vi "DualSimpleLiveAppStreamSaving.vi"() -> ()   [LabVIEW 2020]
uses:
  C:/Users/Public/Documents/Photometrics/PMQI-LabViewSamples/Examples/2018/Dependencies/PVCamNET.dll
  Dependencies/PVCamNET.dll
panel:
  out "Multi Page TIFF Size Read 2":u64 max=1 step=1
  out "Multi Page TIFF Size Read":u64 max=1 step=1
  in  "Multi Page TIFF Size 2 [B]":u64 max=1 step=1
  out "Big TIFF 2":bool
  in  "Big TIFF On/Off 2":bool
  in  "Multi Page TIFF Size [B]":u64 max=1 step=1
  out "Big TIFF":bool
  in  "Big TIFF On/Off":bool
  in  "Trigger Out Behaviour 2":string(combo)
  in  "Trigger In Behaviour 2":string(combo)
  in  "Trigger Out Behaviour":string(combo)
  in  "Trigger In Behaviour":string(combo)
  in  "Live 3":bool
  out "Disk Streaming Queue Size 2":u64
  out "Dropped Frames 2":i32
  out "Buffer Index 2":i32
  in  "Path 2":path
  out "StreamSavingPath 2":string
  in  "Format 2":u8 max=1 step=1
  out "Stream Saving 2":bool
  in  "Stream Saving On/Off 2":bool
  in  "Exposure Time 2":dbl
  in  "Live 2":bool
  out "Available Ram":u64
  out "Disk Streaming Queue Size":u64
  out "Dropped Frames":i32
  out "Buffer Index":i32
  in  "Path":path
  out "StreamSavingPath":string
  in  "Format":u8 max=1 step=1
  out "Stream Saving":bool
  in  "Stream Saving On/Off":bool
  in  "Exposure Time":dbl
  in  "Live":bool
  in  "Camera Status":bool
  in  "Uninit":bool
  in  "Live stop":bool
  in  "Live start":bool
  in  "Init":bool
  # "DualSimpleLiveAppStreamSaving.vi\n\nDescription:\nThis sample code lets the user use \nstream saving and trigger in/out with live mode \nin an event driven structure.\n\nSteps to run:\n1. Connect two cameras. \n2. Click \"Run\"\n3. Click \"Open\" to open two cameras\n4. Enter Exposure Time\n5. Turn On/Off display\n6. Toggle Big TIFF\n7. Enter multi page TIFF size (at default the staxk size is 2GB for regular TIFF and 4GB for Big TIFF)\n8. Select the path for images to be saved at\n9. Turn \"On\" Stream Saving\n10. Click \"Live start\"\n11. Click \"Live stop\"\n12. Click \"Close\""
  # "Camera 1"
  # "Camera 2"
  # "Note about Tiff and BigTiff saving:\n\n\tAt default images are stored with regular Tiff and the maximum multi-image size is 2GB.\n\nIf you would like to save 6GB with Big Tiff then\n    BIG TIFF ON /OFF = ON;\n    Multi Page TIFF Size = 6442450944; (in bytes)\n\t\t\nIfyou would like to save 1 page per file with regular Tiff\n    BIG TIFF ON /OFF = ON;\n    Multi Page TIFF Size =1; (any number smaller than a frame size except 0)\n\t\t\nIf you would like to save 2GB with regular Tiff then\n    BIG TIFF ON /OFF = OFF;\n    Multi Page TIFF Size = 2147483648;"
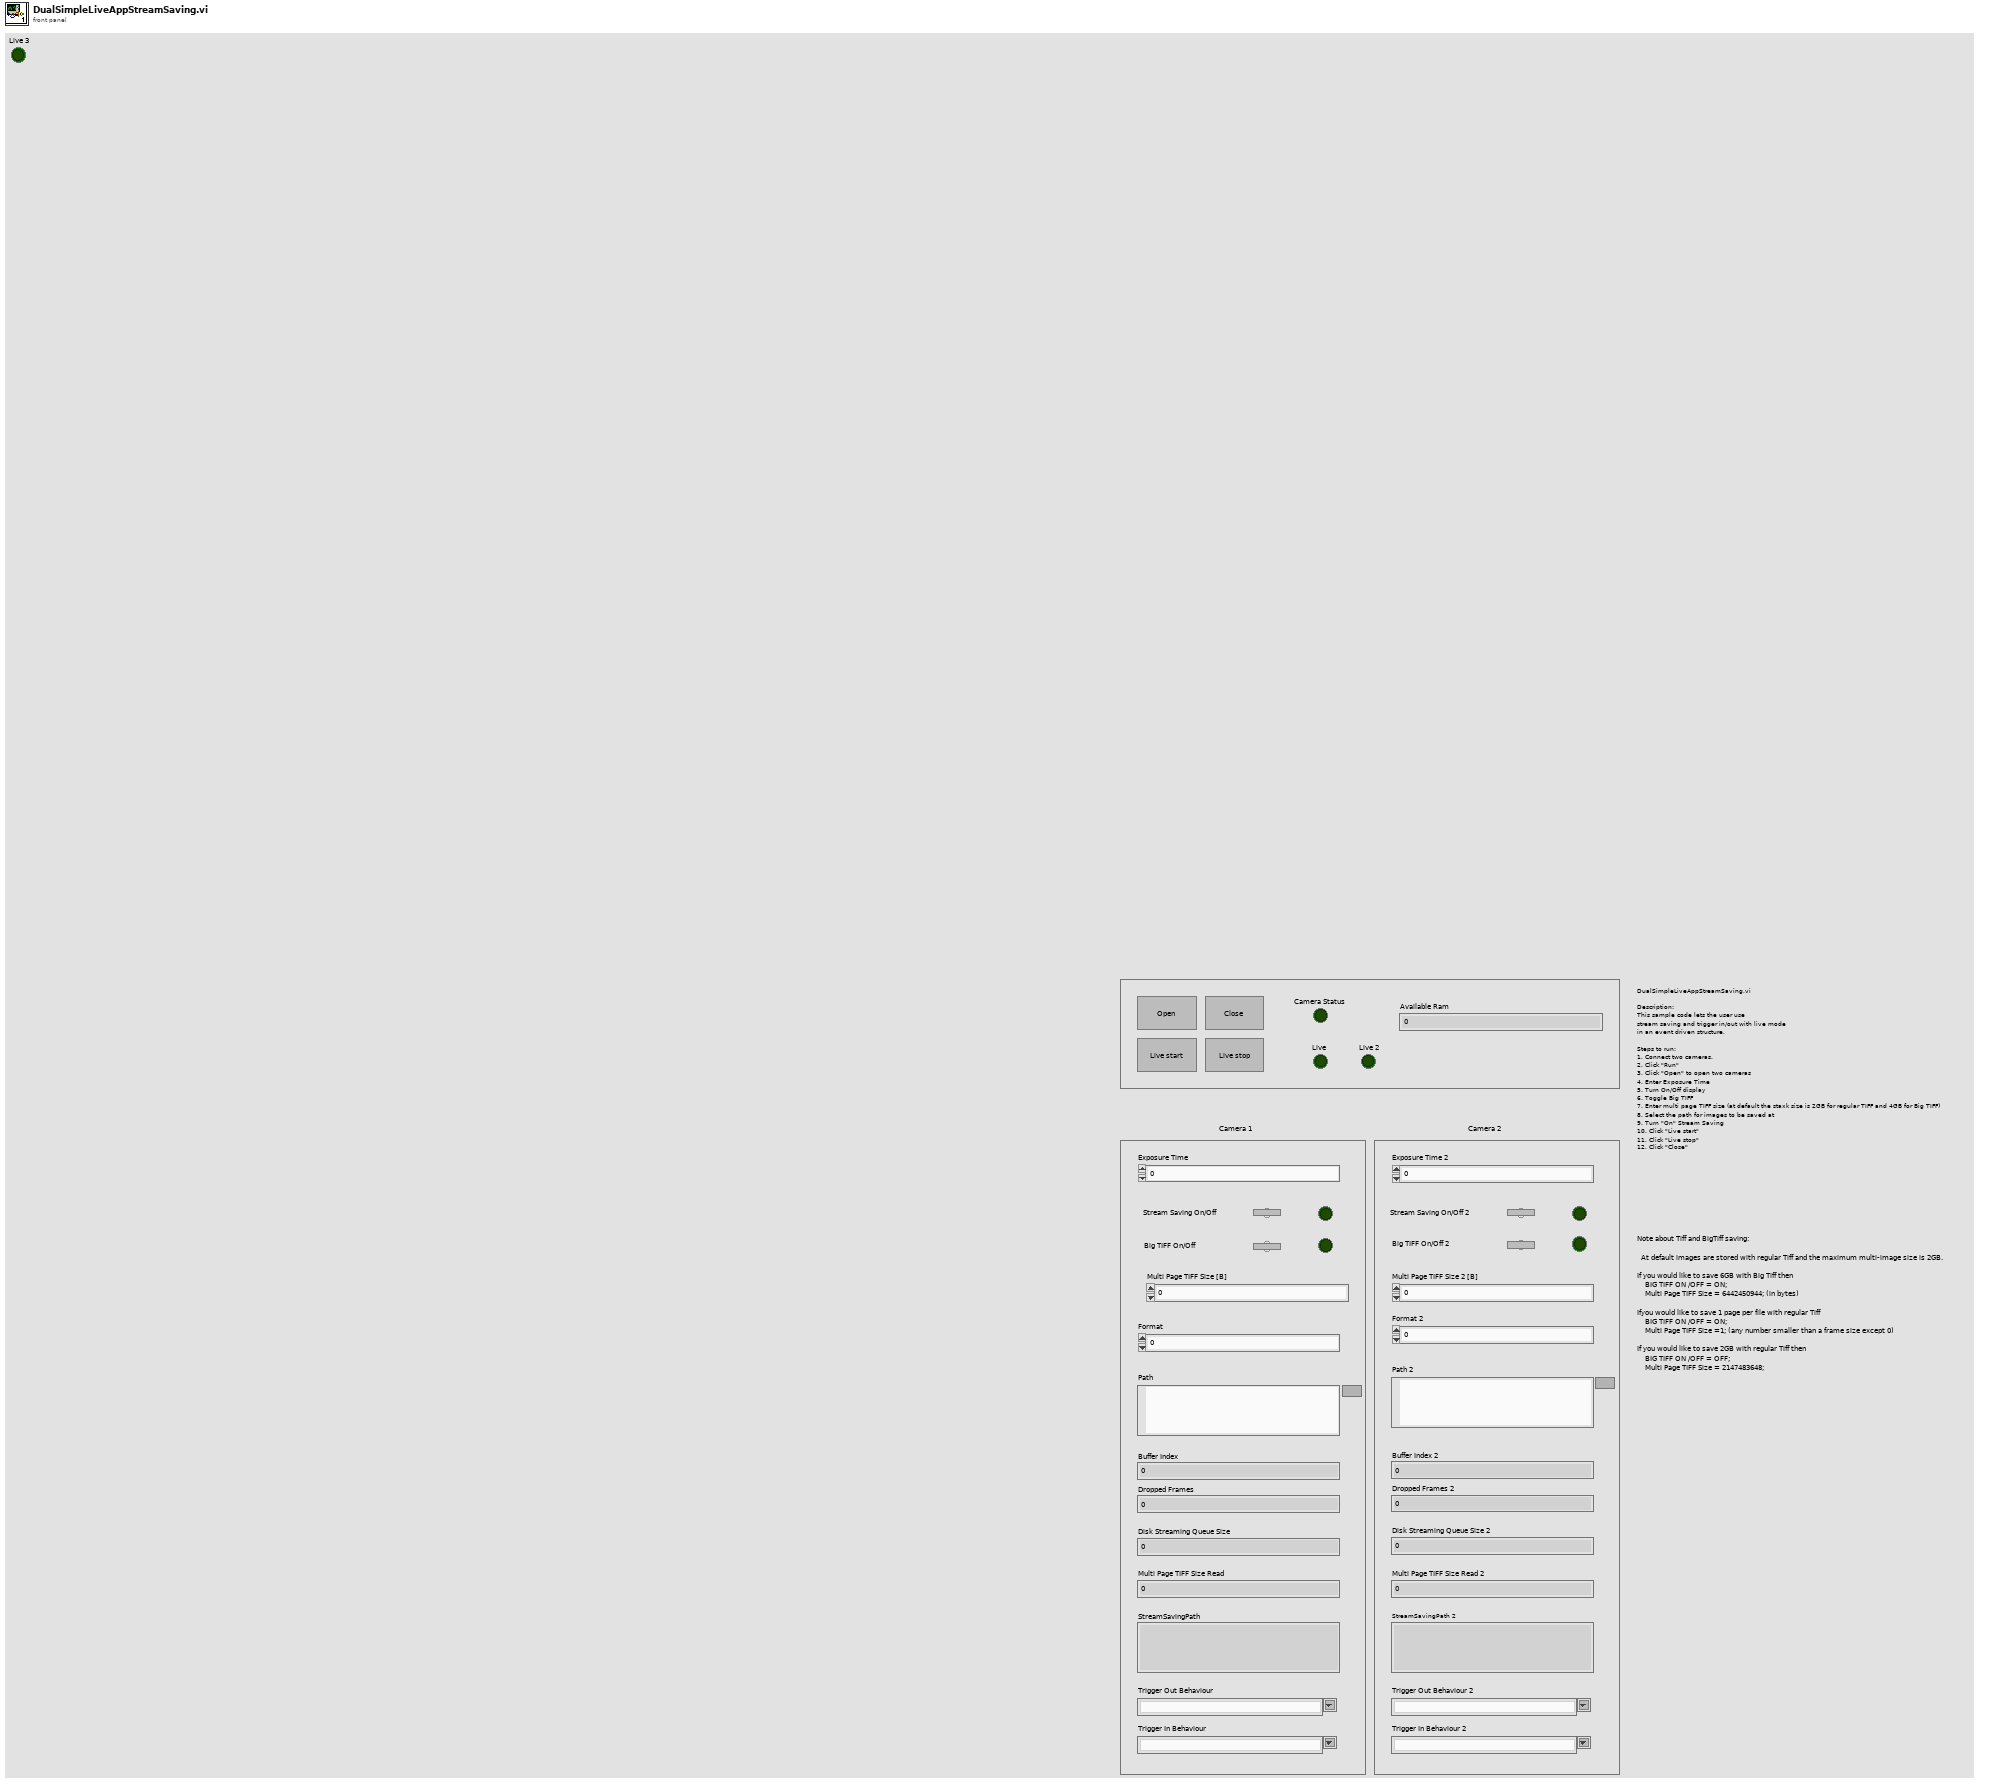
[diagram p1: front panel]
types:
  T1 = cluster{"get_Item":refnum<k24>, "Event Callback":refnum<k27>, "Event Callback":refnum<k27>}
  T2 = cluster{"Disk Streaming Queue Size 2":refnum<vi>, "Dropped Frames 2":refnum<vi>, "Buffer Index 2":refnum<vi>}
  T3 = cluster{"Buffer Index":refnum<vi>, "Dropped Frames":refnum<vi>, "Disk Streaming Queue Size":refnum<vi>, "Available Ram":refnum<vi>}
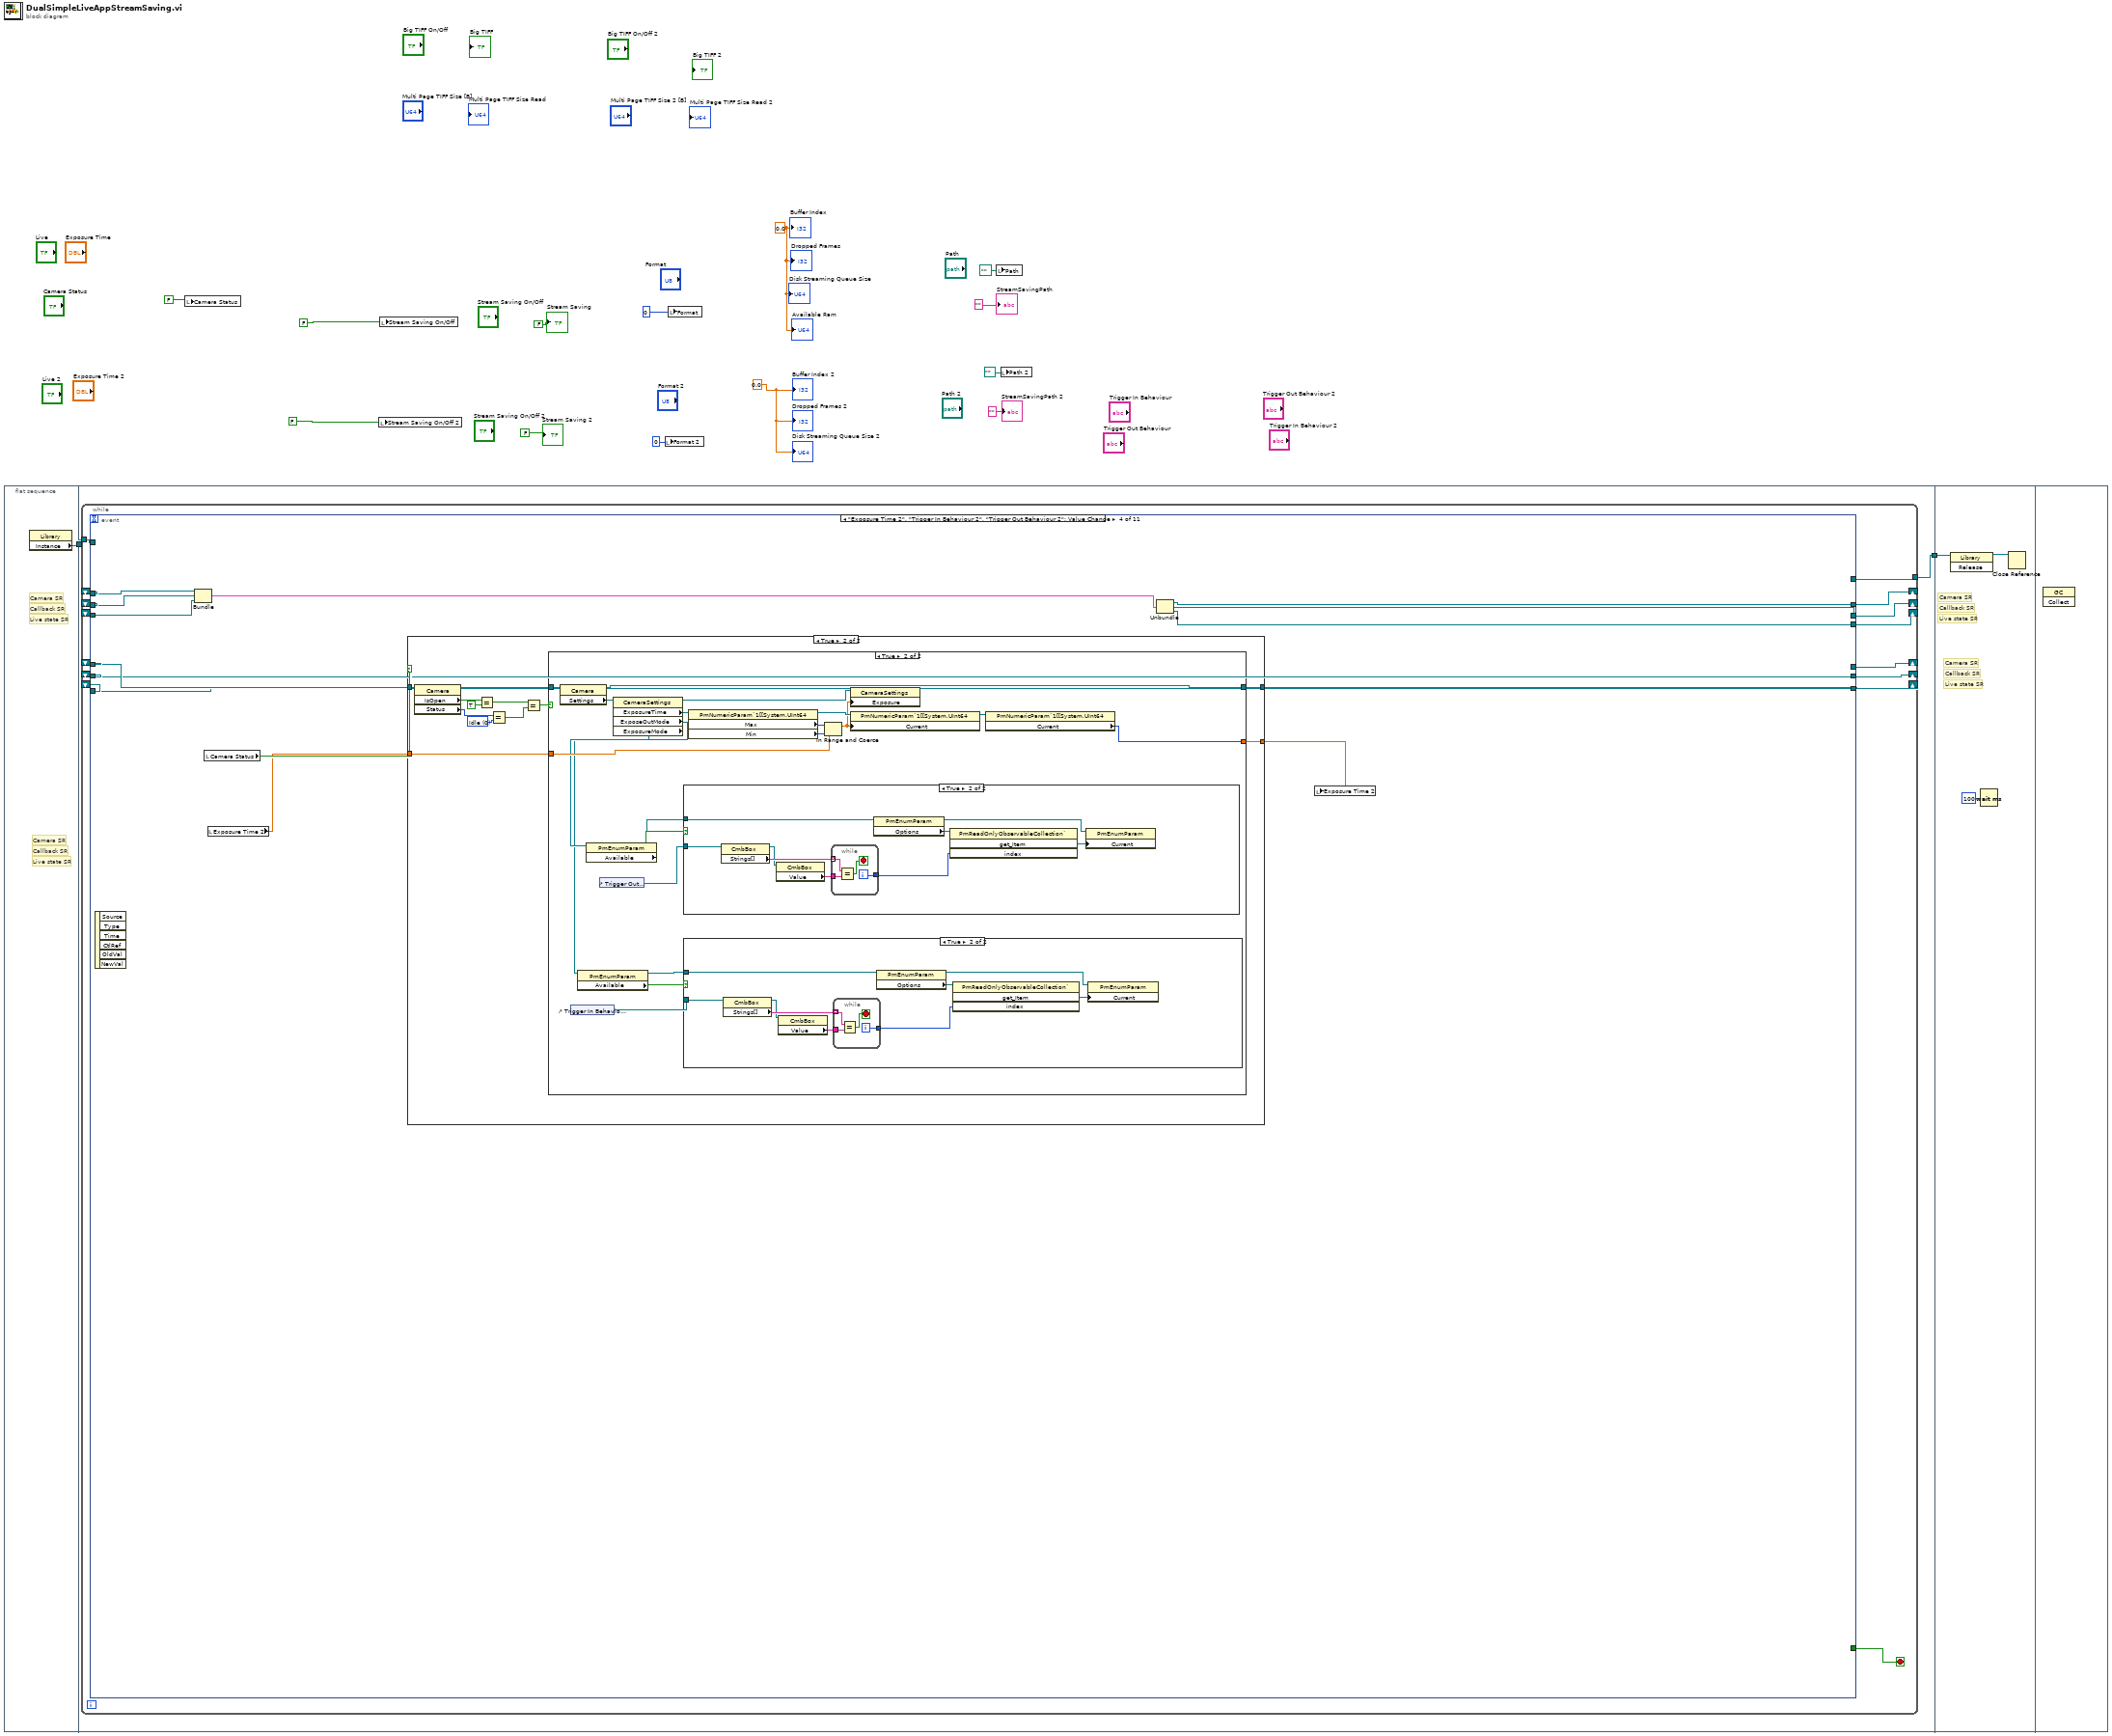
[diagram p0: block diagram]
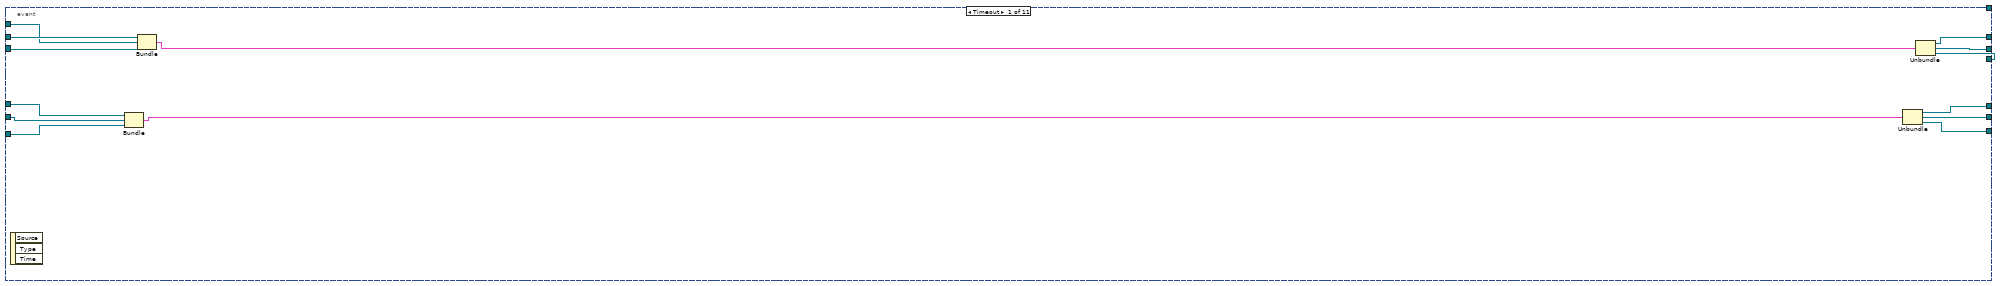
[diagram p2: hidden frame]
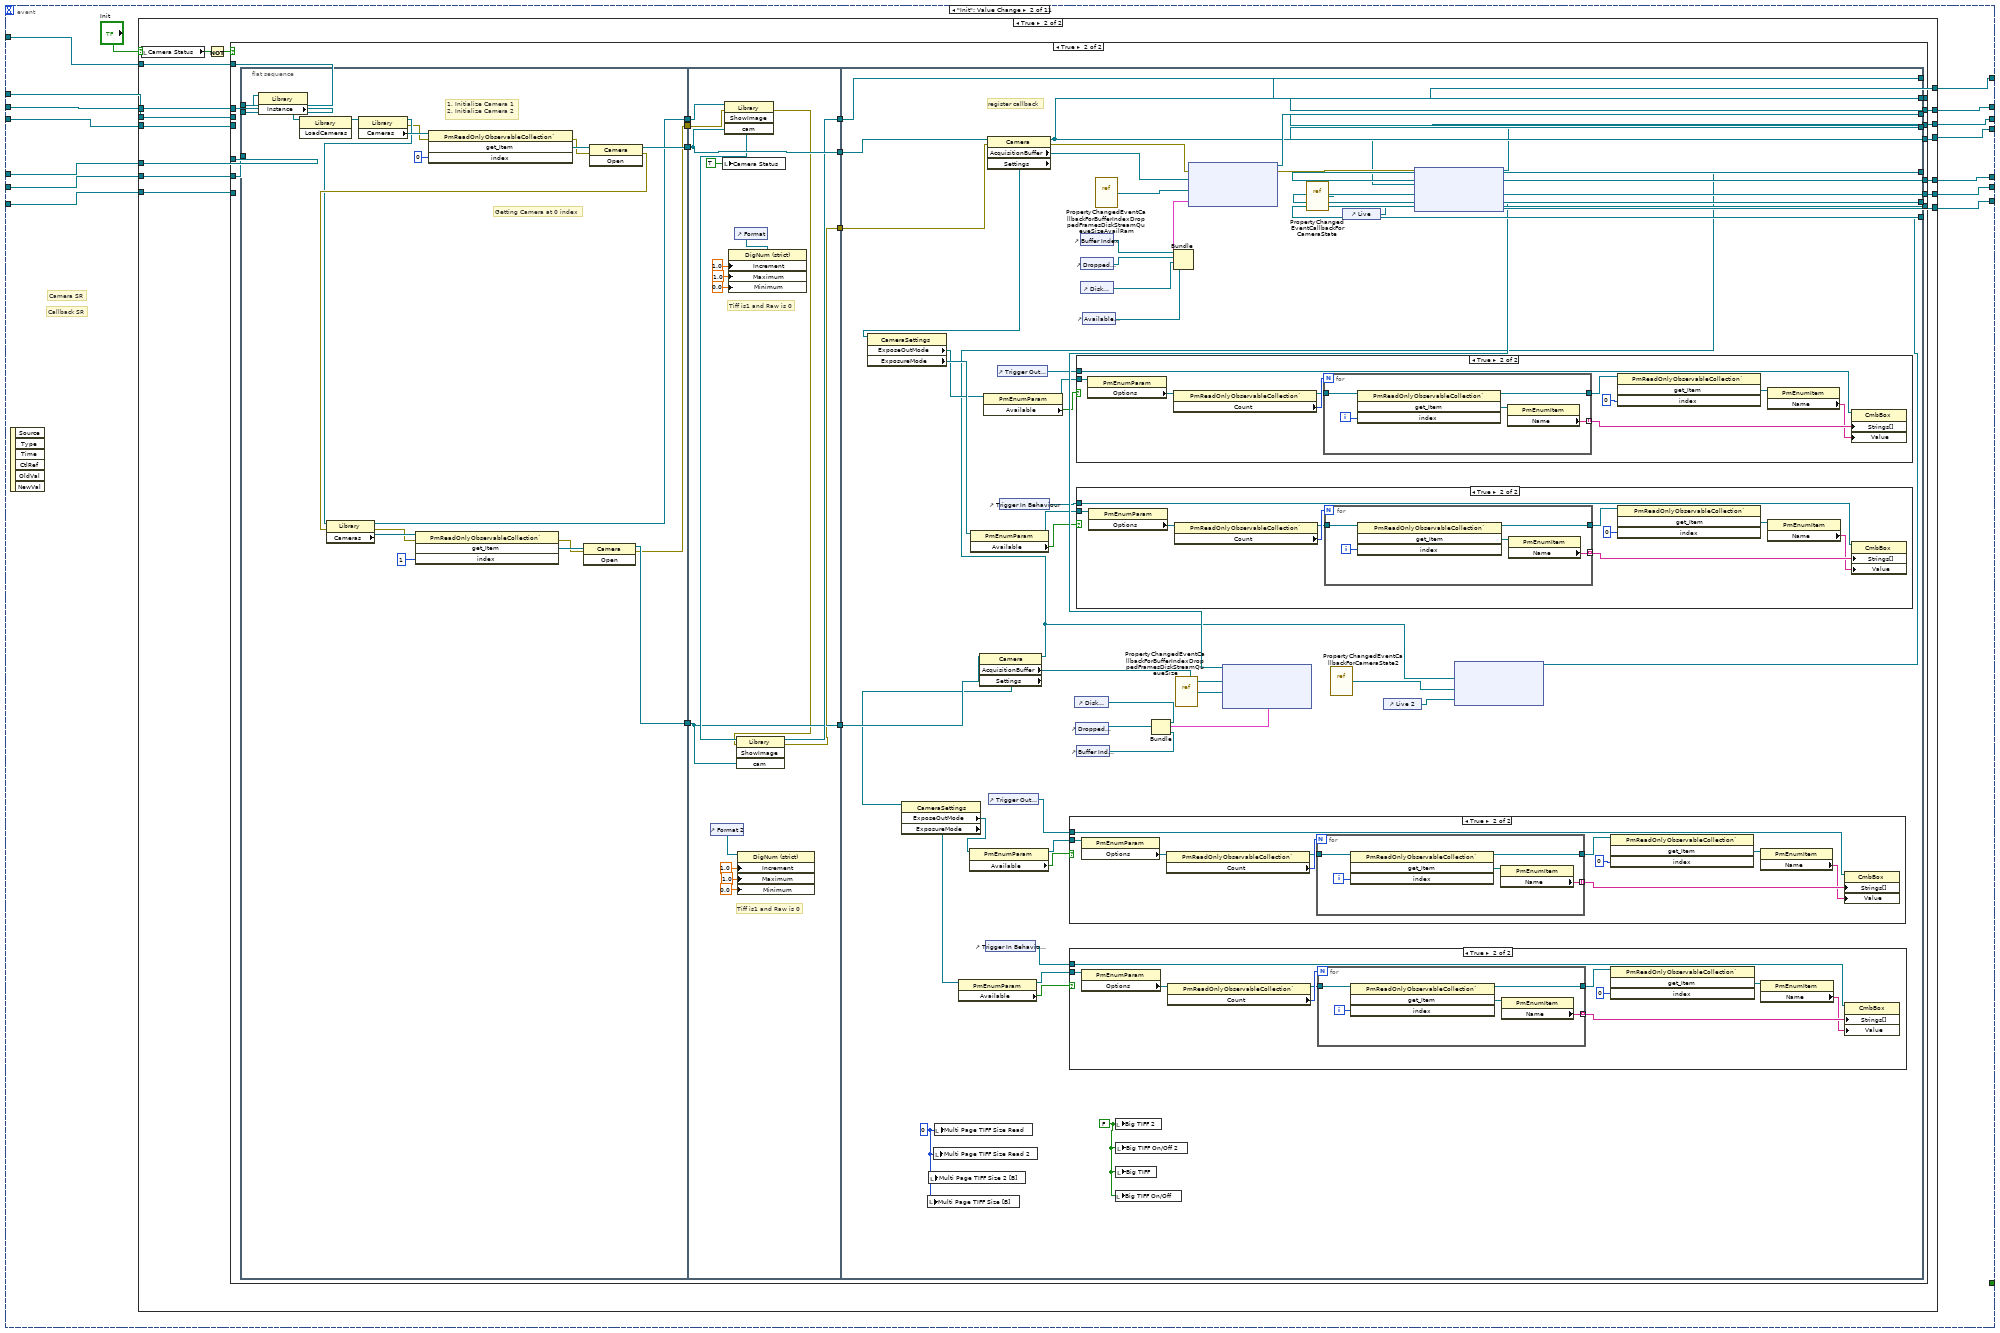
[diagram p3: hidden frame]
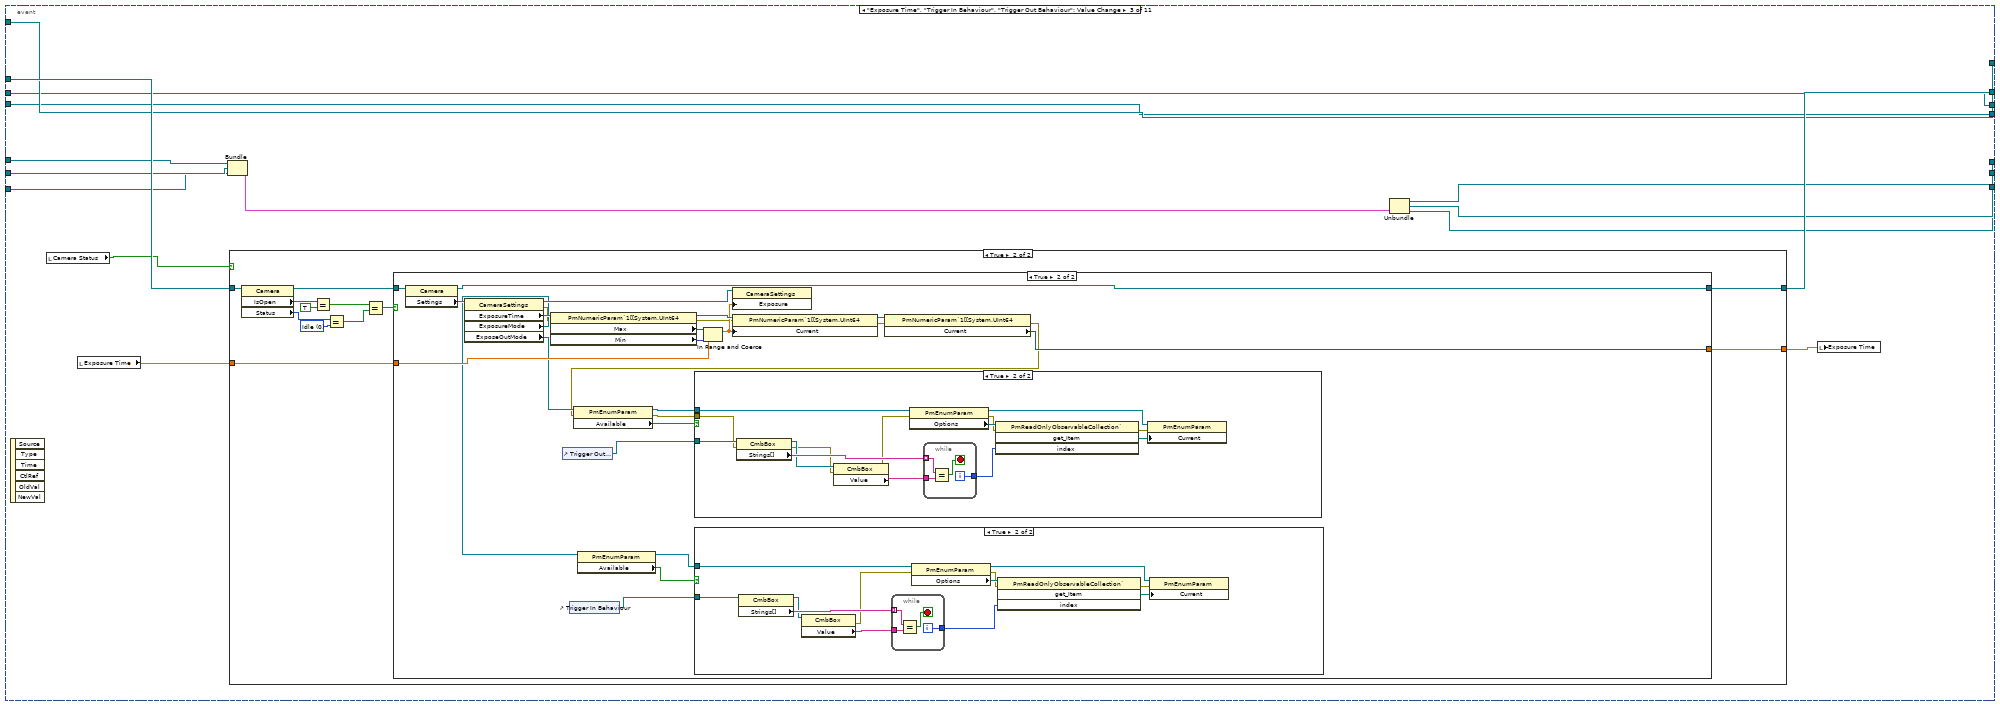
[diagram p10: hidden frame]
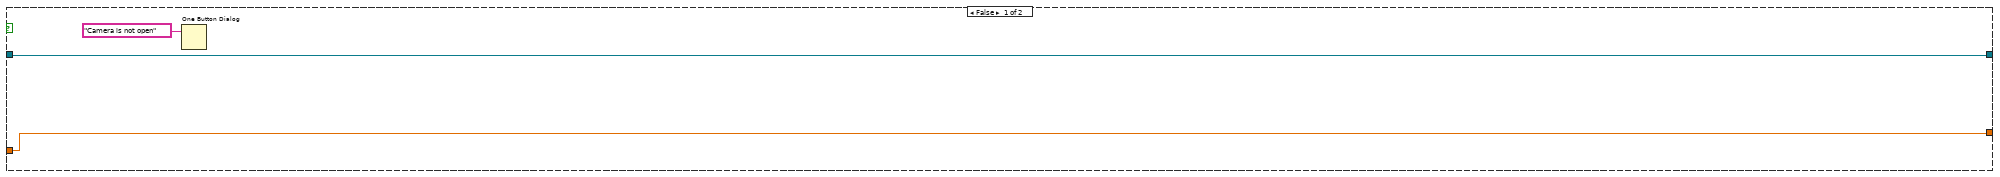
[diagram p11: hidden frame]
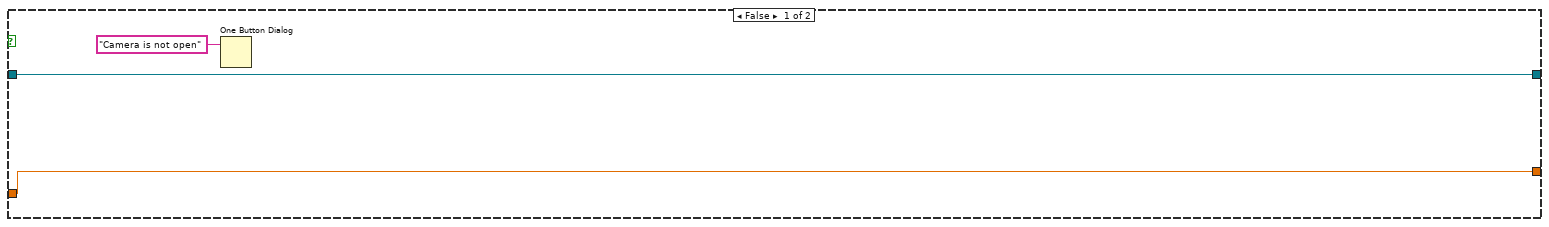
[diagram p15: hidden frame]
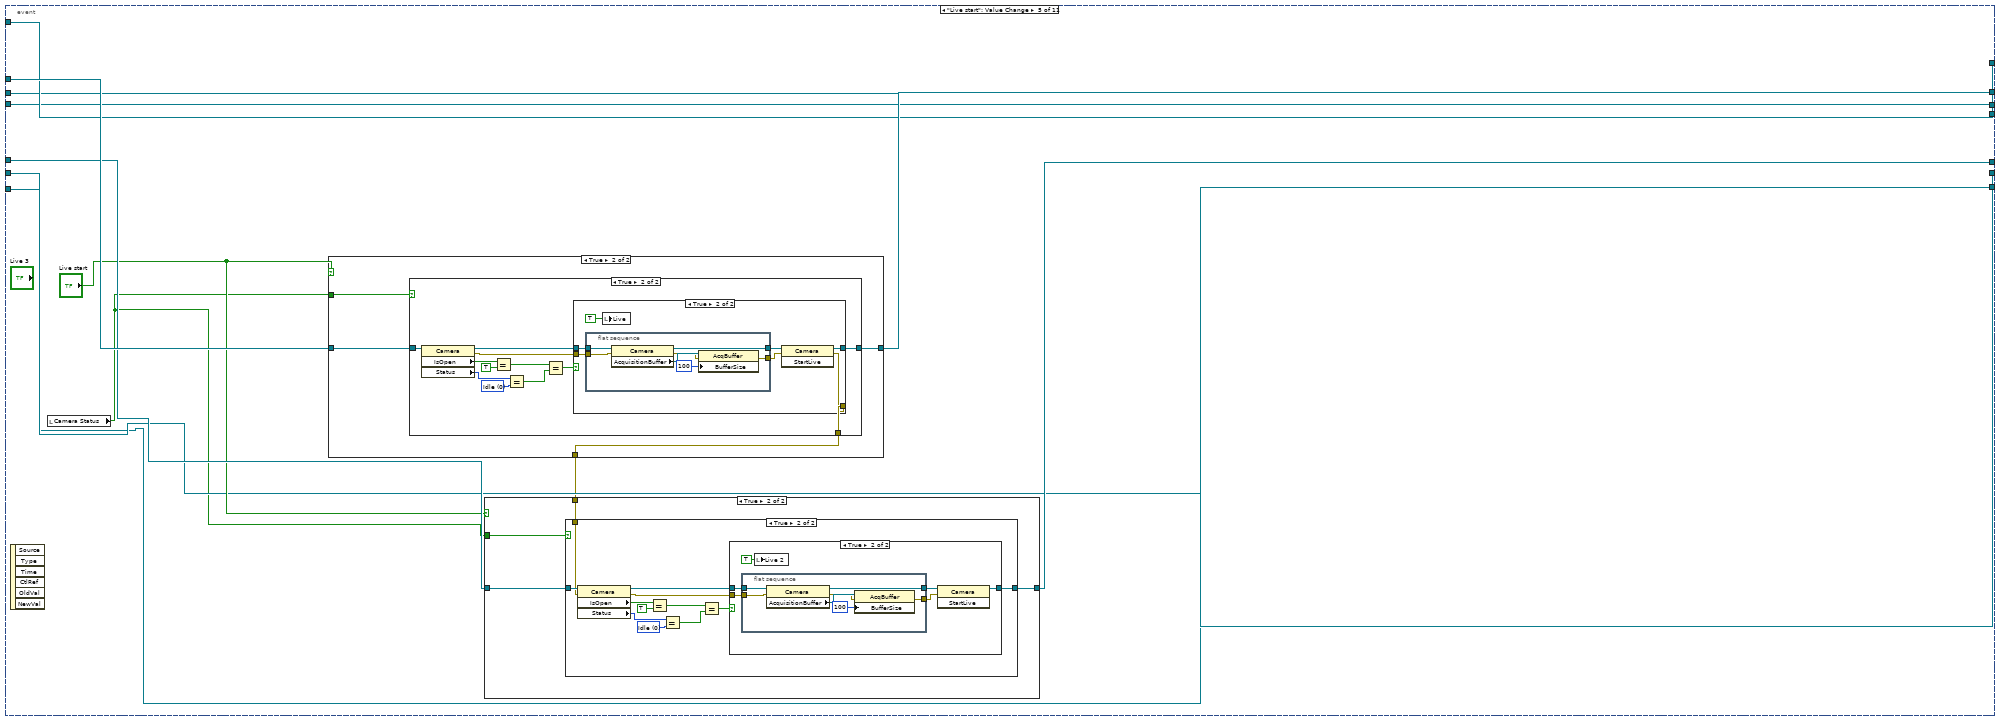
[diagram p19: hidden frame]
diagram:
  w2 = 0.0 ("Buffer Index")
  w7 = 0.0 ("Buffer Index")
  n1 = flat-sequence {
    tunnel: [w16] -> w15
    tunnel: w15 -> [w18]
    tunnel: [w17] -> w14
    tunnel: w14 -> [w898]
    frame #0 {
      # "Live state SR"
      # "Callback SR"
      # "Camera SR"
      # "Live state SR"
      # "Callback SR"
      # "Camera SR"
      n2 = property class="Library"() -> ("Instance"=w16:refnum<k24>)  [unwired: 2 in, 2 out]
    }
    frame #1 {
      n3 = while {
        tunnel: w18 -> [w33]
        shift-right: [w32] -> _
        shift-left: _ -> [w30]
        tunnel: [w31] -> w17
        shift-right: [w28] -> _
        shift-left: _ -> [w27]
        shift-right: [w26] -> _
        shift-left: _ -> [w25]
        shift-right: [w21] -> _
        shift-left: _ -> [w24]
        shift-right: [w20] -> _
        shift-left: _ -> [w22]
        shift-right: [w19] -> _
        shift-left: _ -> [w23]
        stop <- w29 stop-if-true
        n4 = event shown="[3] \"Exposure Time 2\", \"Trigger In Behaviour 2\", \"Trigger Out Behaviour 2\": Value Change" {
          selector: _ -> [_ _ _ _ _ _ _ _ _ _ _]
          dyn-events: _ -> [_ _ _ _ _ _ _ _ _ _ _]
          timeout: _ -> [_ _ _ _ _ _ _ _ _ _ _]
          tunnel: w33 -> [_ w62 w268 _ w434 _ _ _ _ _ w794]
          tunnel: [w39 w61 w270 w350 w435 w525 w579 w649 w685 w730 w795] -> w32
          tunnel: [_ w60 w268 _ w434 _ _ _ _ _ w794] -> w31
          tunnel: w30 -> [w47 w59 w271 w354 w436 w526 w583 w650 w683 w731 w789]
          tunnel: [_ _ _ _ _ _ _ _ _ _ w793] -> w29
          tunnel: [w38 w57 w267 w349 w432 w524 w578 w648 w684 w729 w790] -> w28
          tunnel: w27 -> [w46 w56 w267 w353 w432 w524 w582 w648 w682 w729 w791]
          tunnel: [w37 w55 w266 w348 w433 w523 w577 w647 w680 w728 w788] -> w26
          tunnel: w25 -> [w45 w54 w266 w352 w433 w523 w581 w647 w681 w728 w787]
          tunnel: w24 -> [w44 w53 w263 w361 w430 w517 w593 w645 w690 w726 w784]
          tunnel: w23 -> [w42 w52 w261 w358 w427 w515 w591 w643 w687 w723 w782]
          tunnel: w22 -> [w43 w51 w262 w359 w428 w516 w592 w644 w688 w724 w783]
          tunnel: [w36 w50 w259 w355 w431 w513 w584 w641 w689 w725 w781] -> w21
          tunnel: [w35 w49 w258 w359 w428 w512 w592 w640 w688 w724 w786] -> w20
          tunnel: [w34 w48 w257 w358 w427 w511 w591 w639 w687 w723 w785] -> w19
          event Timeout {
            n5 = event-data() -> ()  [unwired: 1 in, 3 out]
            n6 = Bundle("get_Item"=w44, "Event Callback"=w43, "Event Callback"=w42) -> (w41:T1)  [unwired: 1 in]
            n7 = Bundle("get_Item"=w47, "Event Callback"=w46, "Event Callback"=w45) -> (w40:T1)  [unwired: 1 in]
            n8 = Unbundle(w41) -> ("get_Item"=w36:refnum<k24>, "Event Callback"=w35:refnum<k27>, "Event Callback"=w34:refnum<k27>)
            n9 = Unbundle(w40) -> ("get_Item"=w39:refnum<k24>, "Event Callback"=w38:refnum<k27>, "Event Callback"=w37:refnum<k27>)
          }
          event "Init": Value Change {
            # "Camera SR"
            # "Callback SR"
            n10 = event-data() -> ()  [unwired: 1 in, 6 out]
            n11 = case shown="True" "Init" {
              tunnel: w62 -> [w69 w85]
              tunnel: [w68 w84] -> w61
              tunnel: [w69 w78] -> w60
              tunnel: w59 -> [w68 w81]
              tunnel: [w67 w79] -> w57
              tunnel: w56 -> [w67 w80]
              tunnel: [w66 w77] -> w55
              tunnel: w54 -> [w66 w76]
              tunnel: w53 -> [w65 w75]
              tunnel: w52 -> [w63 w74]
              tunnel: w51 -> [w64 w73]
              tunnel: [w65 w72] -> w50
              tunnel: [w64 w71] -> w49
              tunnel: [w63 w70] -> w48
              frame False {
              }
              frame True {
                n12 = local read "Camera Status"() -> (w83:bool)
                n13 = Not(x=w83) -> (.not. x?=w82:bool)
                n14 = case shown="True" w82 {
                  tunnel: w85 -> [w91 w108]
                  tunnel: [w92 w107] -> w84
                  tunnel: [w91 w106] -> w78
                  tunnel: w81 -> [w92 _]
                  tunnel: [w90 w103] -> w79
                  tunnel: w80 -> [w90 w102]
                  tunnel: [w89 w101] -> w77
                  tunnel: w76 -> [w89 _]
                  tunnel: w75 -> [w88 _]
                  tunnel: w74 -> [w86 _]
                  tunnel: w73 -> [w87 w99]
                  tunnel: [w88 w97] -> w72
                  tunnel: [w87 w96] -> w71
                  tunnel: [w86 w95] -> w70
                  frame False {
                  }
                  frame True {
                    n15 = flat-sequence {
                      tunnel: w108 -> [w126]
                      tunnel: [w114] -> w110
                      tunnel: [w127] -> w109
                      tunnel: w102 -> [_]
                      tunnel: [w113] -> w100
                      tunnel: [w112] -> _
                      tunnel: w99 -> [w112]
                      tunnel: [w111] -> w94
                      tunnel: w110 -> [w146]
                      tunnel: w109 -> [w147]
                      tunnel: [w147] -> w105
                      tunnel: [w139] -> w104
                      tunnel: w100 -> [w134]
                      tunnel: [w134] -> w98
                      tunnel: w94 -> [w133]
                      tunnel: [w131] -> w93
                      tunnel: [w196] -> w106
                      tunnel: [w151] -> w107
                      tunnel: w105 -> [w190]
                      tunnel: w104 -> [w196]
                      tunnel: [w186] -> w103
                      tunnel: [w187] -> w101
                      tunnel: w98 -> [w179]
                      tunnel: [w150] -> w97
                      tunnel: [w181] -> w96
                      tunnel: [w177] -> w95
                      tunnel: w93 -> [w154]
                      frame #0 {
                        # "1. Initialize Camera 1 \n2. Initialize Camera 2"
                        # "Getting Camera at 0 index"
                        n16 = property class="Library"(reference=w126) -> ("Instance"=w125:refnum<k24>)  [unwired: 1 in, 2 out]
                        n17 = invoke class="Library" method="LoadCameras"(reference=w125) -> (reference out=w124:refnum<k24>)  [unwired: 2 in, 2 out]
                        n18 = property class="Library"(reference=w124) -> (reference out=w117:refnum<k24>, error out=w116:errorcluster, "Cameras"=w130:refnum<k24>)  [unwired: 1 in]
                        n19 = invoke class="PmReadOnlyObservableCollection`" method="get_Item"(reference=w130, error in=w116, "index"=0) -> (error out=w115:errorcluster, "get_Item"=w128:refnum<k24>)  [unwired: 1 in, 2 out]
                        n20 = invoke class="Camera" method="Open"(reference=w128, error in=w115) -> (reference out=w127:refnum<k24>, error out=w118:errorcluster)  [unwired: 1 in, 1 out]
                        n21 = property class="Library"(reference=w117, error in=w118) -> (reference out=w114:refnum<k24>, error out=w120:errorcluster, "Cameras"=w123:refnum<k24>)
                        n22 = invoke class="PmReadOnlyObservableCollection`" method="get_Item"(reference=w123, error in=w120, "index"=1) -> (error out=w119:errorcluster, "get_Item"=w121:refnum<k24>)  [unwired: 1 in, 2 out]
                        n23 = invoke class="Camera" method="Open"(reference=w121, error in=w119) -> (reference out=w113:refnum<k24>, error out=w111:errorcluster)  [unwired: 1 in, 1 out]
                      }
                      frame #1 {
                        # "Tiff is1 and Raw is 0"
                        # "Tiff is1 and Raw is 0"
                        n24 = control-ref of="Format 2"() -> (w135:refnum<vi>)
                        n25 = local write "Camera Status"(TRUE ("Camera Status")) -> ()
                        n26 = invoke class="Library" method="ShowImage"(reference=w146, error in=w133, "cam"=w147) -> (reference out=w140:refnum<k24>, error out=w132:errorcluster)  [unwired: 1 in, 2 out]
                        n27 = control-ref of="Format"() -> (w144:refnum<vi>)
                        n28 = property class="DigNum (strict)"(reference=w144, "Increment"=1.0 ("Data Entry Limits:Increment"), "Maximum"=1.0 ("Data Entry Limits:Maximum"), "Minimum"=0.0 ("Data Entry Limits:Minimum")) -> ()  [unwired: 1 in, 2 out]
                        n29 = invoke class="Library" method="ShowImage"(reference=w140, error in=w132, "cam"=w134) -> (reference out=w139:refnum<k24>, error out=w131:errorcluster)  [unwired: 1 in, 2 out]
                        n30 = property class="DigNum (strict)"(reference=w135, "Increment"=1.0 ("Data Entry Limits:Increment"), "Maximum"=1.0 ("Data Entry Limits:Maximum"), "Minimum"=0.0 ("Data Entry Limits:Minimum")) -> ()  [unwired: 1 in, 2 out]
                      }
                      frame #2 {
                        w148 = FALSE ("Big TIFF 2")
                        w149 = u64 0 ("Multi Page TIFF Size Read")
                        # "register callback"
                        n31 = local write "Multi Page TIFF Size [B]"(w149) -> ()
                        n32 = local write "Multi Page TIFF Size 2 [B]"(w149) -> ()
                        n33 = local write "Multi Page TIFF Size Read 2"(w149) -> ()
                        n34 = local write "Multi Page TIFF Size Read"(w149) -> ()
                        n35 = property class="Camera"(reference=w179) -> (reference out=w150:refnum<k24>, "AcquisitionBuffer"=w183:refnum<k24>, "Settings"=w155:refnum<k24>)  [unwired: 1 in, 1 out]
                        n36 = property class="CameraSettings"(reference=w155) -> ("ExposeOutMode"=w162:refnum<k24>, "ExposureMode"=w163:refnum<k24>)  [unwired: 1 in, 2 out]
                        n37 = property class="PmEnumParam"(reference=w163) -> (reference out=w158:refnum<k24>, "Available"=w160:bool)  [unwired: 1 in, 1 out]
                        n38 = property class="PmEnumParam"(reference=w162) -> (reference out=w159:refnum<k24>, "Available"=w161:bool)  [unwired: 1 in, 1 out]
                        n39 = control-ref of="Trigger In Behaviour 2"() -> (w156:refnum<vi>)
                        n40 = property class="Camera"(reference=w190, error in=w154) -> (reference out=w151:refnum<k24>, error out=w153:errorcluster, "AcquisitionBuffer"=w191:refnum<k24>, "Settings"=w164:refnum<k24>)
                        n41 = property class="CameraSettings"(reference=w164) -> ("ExposeOutMode"=w165:refnum<k24>, "ExposureMode"=w166:refnum<k24>)  [unwired: 1 in, 2 out]
                        n42 = property class="PmEnumParam"(reference=w166) -> (reference out=w170:refnum<k24>, "Available"=w171:bool)  [unwired: 1 in, 1 out]
                        n43 = property class="PmEnumParam"(reference=w165) -> (reference out=w169:refnum<k24>, "Available"=w172:bool)  [unwired: 1 in, 1 out]
                        n44 = control-ref of="Trigger Out Behaviour 2"() -> (w157:refnum<vi>)
                        n45 = control-ref of="Trigger Out Behaviour"() -> (w167:refnum<vi>)
                        n46 = control-ref of="Trigger In Behaviour"() -> (w168:refnum<vi>)
                        n47 = case shown="True" w161 {
                          tunnel: w159 -> [_ w221]
                          tunnel: w157 -> [_ w212]
                          frame False {
                          }
                          frame True {
                            n48 = property class="PmEnumParam"(reference=w221) -> ("Options"=w220:refnum<k24>)  [unwired: 1 in, 2 out]
                            n49 = property class="PmReadOnlyObservableCollection`"(reference=w220) -> (reference out=w218:refnum<k24>, "Count"=w219:i32)  [unwired: 1 in, 1 out]
                            n50 = for {
                              N: w219 -> [_]
                              tunnel: w218 -> [w226]
                              tunnel: [w223] -> w215
                              tunnel: [w222] -> w214 mode=indexing
                              i -> [w225]
                              n51 = invoke class="PmReadOnlyObservableCollection`" method="get_Item"(reference=w226, "index"=w225) -> (reference out=w223:refnum<k24>, "get_Item"=w224:refnum<k24>)  [unwired: 2 in, 2 out]
                              n52 = property class="PmEnumItem"(reference=w224) -> ("Name"=w222:string)  [unwired: 1 in, 2 out]
                            }
                            n53 = invoke class="PmReadOnlyObservableCollection`" method="get_Item"(reference=w215, "index"=0) -> ("get_Item"=w216:refnum<k24>)  [unwired: 2 in, 3 out]
                            n54 = property class="PmEnumItem"(reference=w216) -> ("Name"=w213:string)  [unwired: 1 in, 2 out]
                            n55 = property class="CmbBox"(reference=w212, "Strings[]"=w214, "Value"=w213) -> ()  [unwired: 1 in, 2 out]
                          }
                        }
                        n56 = case shown="True" w160 {
                          tunnel: w158 -> [_ w206]
                          tunnel: w156 -> [_ w197]
                          frame False {
                          }
                          frame True {
                            n57 = property class="PmEnumParam"(reference=w206) -> ("Options"=w205:refnum<k24>)  [unwired: 1 in, 2 out]
                            n58 = property class="PmReadOnlyObservableCollection`"(reference=w205) -> (reference out=w203:refnum<k24>, "Count"=w204:i32)  [unwired: 1 in, 1 out]
                            n59 = for {
                              N: w204 -> [_]
                              tunnel: w203 -> [w211]
                              tunnel: [w208] -> w202
                              tunnel: [w207] -> w199 mode=indexing
                              i -> [w210]
                              n60 = invoke class="PmReadOnlyObservableCollection`" method="get_Item"(reference=w211, "index"=w210) -> (reference out=w208:refnum<k24>, "get_Item"=w209:refnum<k24>)  [unwired: 2 in, 2 out]
                              n61 = property class="PmEnumItem"(reference=w209) -> ("Name"=w207:string)  [unwired: 1 in, 2 out]
                            }
                            n62 = invoke class="PmReadOnlyObservableCollection`" method="get_Item"(reference=w202, "index"=0) -> ("get_Item"=w200:refnum<k24>)  [unwired: 2 in, 3 out]
                            n63 = property class="PmEnumItem"(reference=w200) -> ("Name"=w198:string)  [unwired: 1 in, 2 out]
                            n64 = property class="CmbBox"(reference=w197, "Strings[]"=w199, "Value"=w198) -> ()  [unwired: 1 in, 2 out]
                          }
                        }
                        n65 = control-ref of="Disk Streaming Queue Size 2"() -> (w174:refnum<vi>)
                        n66 = control-ref of="Dropped Frames 2"() -> (w175:refnum<vi>)
                        n67 = case shown="True" w172 {
                          tunnel: w169 -> [_ w251]
                          tunnel: w167 -> [_ w242]
                          frame False {
                          }
                          frame True {
                            n68 = property class="PmEnumParam"(reference=w251) -> ("Options"=w250:refnum<k24>)  [unwired: 1 in, 2 out]
                            n69 = property class="PmReadOnlyObservableCollection`"(reference=w250) -> (reference out=w248:refnum<k24>, "Count"=w249:i32)  [unwired: 1 in, 1 out]
                            n70 = for {
                              N: w249 -> [_]
                              tunnel: w248 -> [w256]
                              tunnel: [w253] -> w245
                              tunnel: [w252] -> w244 mode=indexing
                              i -> [w255]
                              n71 = invoke class="PmReadOnlyObservableCollection`" method="get_Item"(reference=w256, "index"=w255) -> (reference out=w253:refnum<k24>, "get_Item"=w254:refnum<k24>)  [unwired: 2 in, 2 out]
                              n72 = property class="PmEnumItem"(reference=w254) -> ("Name"=w252:string)  [unwired: 1 in, 2 out]
                            }
                            n73 = invoke class="PmReadOnlyObservableCollection`" method="get_Item"(reference=w245, "index"=0) -> ("get_Item"=w246:refnum<k24>)  [unwired: 2 in, 3 out]
                            n74 = property class="PmEnumItem"(reference=w246) -> ("Name"=w243:string)  [unwired: 1 in, 2 out]
                            n75 = property class="CmbBox"(reference=w242, "Strings[]"=w244, "Value"=w243) -> ()  [unwired: 1 in, 2 out]
                          }
                        }
                        n76 = control-ref of="Buffer Index 2"() -> (w173:refnum<vi>)
                        n77 = case shown="True" w171 {
                          tunnel: w170 -> [_ w236]
                          tunnel: w168 -> [_ w227]
                          frame False {
                          }
                          frame True {
                            n78 = property class="PmEnumParam"(reference=w236) -> ("Options"=w235:refnum<k24>)  [unwired: 1 in, 2 out]
                            n79 = property class="PmReadOnlyObservableCollection`"(reference=w235) -> (reference out=w233:refnum<k24>, "Count"=w234:i32)  [unwired: 1 in, 1 out]
                            n80 = for {
                              N: w234 -> [_]
                              tunnel: w233 -> [w241]
                              tunnel: [w238] -> w232
                              tunnel: [w237] -> w229 mode=indexing
                              i -> [w240]
                              n81 = invoke class="PmReadOnlyObservableCollection`" method="get_Item"(reference=w241, "index"=w240) -> (reference out=w238:refnum<k24>, "get_Item"=w239:refnum<k24>)  [unwired: 2 in, 2 out]
                              n82 = property class="PmEnumItem"(reference=w239) -> ("Name"=w237:string)  [unwired: 1 in, 2 out]
                            }
                            n83 = invoke class="PmReadOnlyObservableCollection`" method="get_Item"(reference=w232, "index"=0) -> ("get_Item"=w230:refnum<k24>)  [unwired: 2 in, 3 out]
                            n84 = property class="PmEnumItem"(reference=w230) -> ("Name"=w228:string)  [unwired: 1 in, 2 out]
                            n85 = property class="CmbBox"(reference=w227, "Strings[]"=w229, "Value"=w228) -> ()  [unwired: 1 in, 2 out]
                          }
                        }
                        n86 = control-ref of="Buffer Index"() -> (w195:refnum<vi>)
                        n87 = control-ref of="Dropped Frames"() -> (w194:refnum<vi>)
                        n88 = control-ref of="Disk Streaming Queue Size"() -> (w193:refnum<vi>)
                        n89 = control-ref of="Available Ram"() -> (w185:refnum<vi>)
                        n90 = vi-ref "PropertyChangedEventCallbackForBufferIndexDroppedFramesDiskStreamQueueSizeAvailRam.vi"() -> ("vi reference"=w184:refnum<vi>)
                        n91 = local write "Big TIFF 2"(w148) -> ()
                        n92 = local write "Big TIFF On/Off"(w148) -> ()
                        n93 = local write "Big TIFF On/Off 2"(w148) -> ()
                        n94 = local write "Big TIFF"(w148) -> ()
                        n95 = Bundle("Disk Streaming Queue Size 2"=w174, "Dropped Frames 2"=w175, "Buffer Index 2"=w173) -> (w182:T2)  [unwired: 1 in]
                        n96 = Bundle("Buffer Index"=w195, "Dropped Frames"=w194, "Disk Streaming Queue Size"=w193, "Available Ram"=w185) -> (w192:T3)  [unwired: 1 in]
                        n97 = vi-ref "PropertyChangedEventCallbackForBufferIndexDroppedFramesDiskStreamQueueSize.vi"() -> ("vi reference"=w176:refnum<vi>)
                        n98 = node(w153, w191, w184, w192) -> (w186:refnum<k27>, w152:errorcluster)  [unwired: 1 in]
                        n99 = node(w183, w176, w182) -> (w181:refnum<k27>)  [unwired: 2 in, 1 out]
                        n100 = vi-ref "PropertyChangedEventCallbackForCameraState.vi"() -> ("vi reference"=w189:refnum<vi>)
                        n101 = vi-ref "PropertyChangedEventCallbackForCameraState2.vi"() -> ("vi reference"=w178:refnum<vi>)
                        n102 = control-ref of="Live"() -> (w188:refnum<vi>)
                        n103 = control-ref of="Live 2"() -> (w180:refnum<vi>)
                        n104 = node(w152, w151, w189, w188) -> (w187:refnum<k27>)  [unwired: 1 in, 1 out]
                        n105 = node(w150, w178, w180) -> (w177:refnum<k27>)  [unwired: 2 in, 1 out]
                      }
                    }
                  }
                }
              }
            }
          }
          event "Exposure Time", "Trigger In Behaviour", "Trigger Out Behaviour": Value Change {
            n106 = event-data() -> ()  [unwired: 1 in, 6 out]
            n107 = local read "Camera Status"() -> (w269:bool)
            n108 = local read "Exposure Time"() -> (w264:dbl)
            n109 = Bundle("get_Item"=w263, "Event Callback"=w262, "Event Callback"=w261) -> (w260:T1)  [unwired: 1 in]
            n110 = case shown="True" w269 {
              tunnel: w271 -> [w274 w280]
              tunnel: [w274 w277] -> w270
              tunnel: [w272 w276] -> w265
              tunnel: w264 -> [w272 w275]
              frame False {
                n111 = One Button Dialog(message="Camera is not open") -> ()  [unwired: 1 in, 1 out]
              }
              frame True {
                w285 = 0 items=["Idle", "Capturing"] ("Status")
                n112 = property class="Camera"(reference=w280) -> (reference out=w278:refnum<k24>, "IsOpen"=w284:bool, "Status"=w286:i32)  [unwired: 1 in, 1 out]
                n113 = Equal?(x=w284, y=TRUE) -> (x = y?=w282:bool)
                n114 = Equal?(x=w286, y=w285) -> (x = y?=w281:bool)
                n115 = Equal?(x=w282, y=w281) -> (x = y?=w279:bool)
                n116 = case shown="True" w279 {
                  tunnel: w278 -> [w288 w313]
                  tunnel: [w288 w304] -> w277
                  tunnel: [w287 w303] -> w276
                  tunnel: w275 -> [w287 w302]
                  frame False {
                  }
                  frame True {
                    n117 = property class="Camera"(reference=w313) -> (reference out=w304:refnum<k24>, "Settings"=w312:refnum<k24>)  [unwired: 1 in, 1 out]
                    n118 = property class="CameraSettings"(reference=w312) -> (reference out=w305:refnum<k24>, error out=w293:errorcluster, "ExposureTime"=w306:refnum<k24>, "ExposureMode"=w294:refnum<k24>, "ExposeOutMode"=w295:refnum<k24>)  [unwired: 1 in]
                    n119 = property class="PmNumericParam`1[[System.UInt64"(reference=w306, error in=w293) -> (reference out=w309:refnum<k24>, error out=w292:errorcluster, "Max"=w311:u64, "Min"=w310:u64)
                    n120 = control-ref of="Trigger Out Behaviour"() -> (w297:refnum<vi>)
                    n121 = control-ref of="Trigger In Behaviour"() -> (w296:refnum<vi>)
                    n122 = property class="PmEnumParam"(reference=w294) -> (reference out=w299:refnum<k24>, "Available"=w300:bool)  [unwired: 1 in, 1 out]
                    n123 = case shown="True" w300 {
                      tunnel: w299 -> [_ w324]
                      tunnel: w296 -> [_ w317]
                      frame False {
                      }
                      frame True {
                        n124 = property class="CmbBox"(reference=w317) -> (reference out=w319:refnum<vi>, "Strings[]"=w325:string[])  [unwired: 1 in, 1 out]
                        n125 = property class="CmbBox"(reference=w319) -> (error out=w314:errorcluster, "Value"=w318:string)  [unwired: 1 in, 1 out]
                        n126 = while {
                          tunnel: w325 -> [w329] mode=indexing
                          tunnel: [w327] -> w322
                          tunnel: w318 -> [w326]
                          i -> [w327]
                          stop <- w328 stop-if-true
                          n127 = Equal?(x=w329, y=w326) -> (x = y?=w328:bool)
                        }
                        n128 = property class="PmEnumParam"(reference=w324, error in=w314) -> (reference out=w321:refnum<k24>, error out=w315:errorcluster, "Options"=w323:refnum<k24>)
                        n129 = invoke class="PmReadOnlyObservableCollection`" method="get_Item"(reference=w323, error in=w315, "index"=w322) -> (error out=w316:errorcluster, "get_Item"=w320:refnum<k24>)  [unwired: 1 in, 2 out]
                        n130 = property class="PmEnumParam"(reference=w321, error in=w316, "Current"=w320) -> ()  [unwired: 2 out]
                      }
                    }
                    n131 = In Range and Coerce(upper limit=w311, x=w302, lower limit=w310) -> (coerced(x)=w307:dbl)  [unwired: 1 out]
                    n132 = property class="CameraSettings"(reference=w305, "Exposure"=w307) -> ()  [unwired: 1 in, 2 out]
                    n133 = property class="PmNumericParam`1[[System.UInt64"(reference=w309, error in=w292, "Current"=w307) -> (reference out=w308:refnum<k24>, error out=w291:errorcluster)
                    n134 = property class="PmNumericParam`1[[System.UInt64"(reference=w308, error in=w291) -> (error out=w290:errorcluster, "Current"=w303:u64)  [unwired: 1 out]
                    n135 = property class="PmEnumParam"(reference=w295, error in=w290) -> (reference out=w298:refnum<k24>, error out=w289:errorcluster, "Available"=w301:bool)
                    n136 = case shown="True" w301 {
                      tunnel: w298 -> [_ w342]
                      tunnel: w297 -> [_ w335]
                      tunnel: w289 -> [_ w334]
                      frame False {
                      }
                      frame True {
                        n137 = property class="CmbBox"(reference=w335, error in=w334) -> (reference out=w337:refnum<vi>, error out=w333:errorcluster, "Strings[]"=w343:string[])
                        n138 = property class="CmbBox"(reference=w337, error in=w333) -> (error out=w332:errorcluster, "Value"=w336:string)  [unwired: 1 out]
                        n139 = property class="PmEnumParam"(reference=w342, error in=w332) -> (reference out=w339:refnum<k24>, error out=w331:errorcluster, "Options"=w341:refnum<k24>)
                        n140 = while {
                          tunnel: w343 -> [w347] mode=indexing
                          tunnel: [w345] -> w340
                          tunnel: w336 -> [w344]
                          i -> [w345]
                          stop <- w346 stop-if-true
                          n141 = Equal?(x=w347, y=w344) -> (x = y?=w346:bool)
                        }
                        n142 = invoke class="PmReadOnlyObservableCollection`" method="get_Item"(reference=w341, error in=w331, "index"=w340) -> (error out=w330:errorcluster, "get_Item"=w338:refnum<k24>)  [unwired: 1 in, 2 out]
                        n143 = property class="PmEnumParam"(reference=w339, error in=w330, "Current"=w338) -> ()  [unwired: 2 out]
                      }
                    }
                  }
                }
              }
            }
            n144 = Unbundle(w260) -> ("get_Item"=w259:refnum<k24>, "Event Callback"=w258:refnum<k27>, "Event Callback"=w257:refnum<k27>)
            n145 = local write "Exposure Time"(w265) -> ()
          }
          event "Exposure Time 2", "Trigger In Behaviour 2", "Trigger Out Behaviour 2": Value Change {
            n146 = event-data() -> ()  [unwired: 1 in, 6 out]
            n147 = Bundle("get_Item"=w354, "Event Callback"=w353, "Event Callback"=w352) -> (w351:T1)  [unwired: 1 in]
            n148 = local read "Camera Status"() -> (w360:bool)
            n149 = local read "Exposure Time 2"() -> (w357:dbl)
            n150 = case shown="True" w360 {
              tunnel: w361 -> [w364 w370]
              tunnel: [w364 w367] -> w355
              tunnel: [w362 w366] -> w356
              tunnel: w357 -> [w362 w365]
              frame False {
                n151 = One Button Dialog(message="Camera is not open") -> ()  [unwired: 1 in, 1 out]
              }
              frame True {
                w375 = 0 items=["Idle", "Capturing"] ("Status")
                n152 = property class="Camera"(reference=w370) -> (reference out=w368:refnum<k24>, "IsOpen"=w374:bool, "Status"=w376:i32)  [unwired: 1 in, 1 out]
                n153 = Equal?(x=w374, y=TRUE) -> (x = y?=w372:bool)
                n154 = Equal?(x=w376, y=w375) -> (x = y?=w371:bool)
                n155 = Equal?(x=w372, y=w371) -> (x = y?=w369:bool)
                n156 = case shown="True" w369 {
                  tunnel: w368 -> [w378 w398]
                  tunnel: [w378 w389] -> w367
                  tunnel: [w377 w388] -> w366
                  tunnel: w365 -> [w377 w387]
                  frame False {
                  }
                  frame True {
                    n157 = property class="Camera"(reference=w398) -> (reference out=w389:refnum<k24>, "Settings"=w397:refnum<k24>)  [unwired: 1 in, 1 out]
                    n158 = control-ref of="Trigger In Behaviour 2"() -> (w382:refnum<vi>)
                    n159 = control-ref of="Trigger Out Behaviour 2"() -> (w381:refnum<vi>)
                    n160 = property class="CameraSettings"(reference=w397) -> (reference out=w390:refnum<k24>, "ExposureTime"=w391:refnum<k24>, "ExposeOutMode"=w380:refnum<k24>, "ExposureMode"=w379:refnum<k24>)  [unwired: 1 in, 1 out]
                    n161 = property class="PmEnumParam"(reference=w379) -> (reference out=w384:refnum<k24>, "Available"=w385:bool)  [unwired: 1 in, 1 out]
                    n162 = property class="PmEnumParam"(reference=w380) -> (reference out=w383:refnum<k24>, "Available"=w386:bool)  [unwired: 1 in, 1 out]
                    n163 = case shown="True" w386 {
                      tunnel: w383 -> [_ w419]
                      tunnel: w381 -> [_ w412]
                      frame False {
                      }
                      frame True {
                        n164 = property class="CmbBox"(reference=w412) -> (reference out=w414:refnum<vi>, "Strings[]"=w420:string[])  [unwired: 1 in, 1 out]
                        n165 = property class="CmbBox"(reference=w414) -> ("Value"=w413:string)  [unwired: 1 in, 2 out]
                        n166 = while {
                          tunnel: w420 -> [w424] mode=indexing
                          tunnel: [w422] -> w417
                          tunnel: w413 -> [w421]
                          i -> [w422]
                          stop <- w423 stop-if-true
                          n167 = Equal?(x=w424, y=w421) -> (x = y?=w423:bool)
                        }
                        n168 = property class="PmEnumParam"(reference=w419) -> (reference out=w416:refnum<k24>, "Options"=w418:refnum<k24>)  [unwired: 1 in, 1 out]
                        n169 = invoke class="PmReadOnlyObservableCollection`" method="get_Item"(reference=w418, "index"=w417) -> ("get_Item"=w415:refnum<k24>)  [unwired: 2 in, 3 out]
                        n170 = property class="PmEnumParam"(reference=w416, "Current"=w415) -> ()  [unwired: 1 in, 2 out]
                      }
                    }
                    n171 = case shown="True" w385 {
                      tunnel: w384 -> [_ w406]
                      tunnel: w382 -> [_ w399]
                      frame False {
                      }
                      frame True {
                        n172 = property class="CmbBox"(reference=w399) -> (reference out=w401:refnum<vi>, "Strings[]"=w407:string[])  [unwired: 1 in, 1 out]
                        n173 = property class="CmbBox"(reference=w401) -> ("Value"=w400:string)  [unwired: 1 in, 2 out]
                        n174 = while {
                          tunnel: w407 -> [w411] mode=indexing
                          tunnel: [w409] -> w404
                          tunnel: w400 -> [w408]
                          i -> [w409]
                          stop <- w410 stop-if-true
                          n175 = Equal?(x=w411, y=w408) -> (x = y?=w410:bool)
                        }
                        n176 = property class="PmEnumParam"(reference=w406) -> (reference out=w403:refnum<k24>, "Options"=w405:refnum<k24>)  [unwired: 1 in, 1 out]
                        n177 = invoke class="PmReadOnlyObservableCollection`" method="get_Item"(reference=w405, "index"=w404) -> ("get_Item"=w402:refnum<k24>)  [unwired: 2 in, 3 out]
                        n178 = property class="PmEnumParam"(reference=w403, "Current"=w402) -> ()  [unwired: 1 in, 2 out]
                      }
                    }
                    n179 = property class="PmNumericParam`1[[System.UInt64"(reference=w391) -> (reference out=w394:refnum<k24>, "Max"=w396:u64, "Min"=w395:u64)  [unwired: 1 in, 1 out]
                    n180 = In Range and Coerce(upper limit=w396, x=w387, lower limit=w395) -> (coerced(x)=w392:dbl)  [unwired: 1 out]
                    n181 = property class="CameraSettings"(reference=w390, "Exposure"=w392) -> ()  [unwired: 1 in, 2 out]
                    n182 = property class="PmNumericParam`1[[System.UInt64"(reference=w394, "Current"=w392) -> (reference out=w393:refnum<k24>)  [unwired: 1 in, 1 out]
                    n183 = property class="PmNumericParam`1[[System.UInt64"(reference=w393) -> ("Current"=w388:u64)  [unwired: 1 in, 2 out]
                  }
                }
              }
            }
            n184 = Unbundle(w351) -> ("get_Item"=w350:refnum<k24>, "Event Callback"=w349:refnum<k27>, "Event Callback"=w348:refnum<k27>)
            n185 = local write "Exposure Time 2"(w356) -> ()
          }
          event "Live start": Value Change {
            n186 = event-data() -> ()  [unwired: 1 in, 6 out]
            n187 = local read "Camera Status"() -> (w426:bool)
            n188 = case shown="True" "Live start" {
              tunnel: w436 -> [w471 w475]
              tunnel: [w471 w474] -> w435
              tunnel: w426 -> [_ w473]
              tunnel: [_ w472] -> w425
              frame False {
              }
              frame True {
                n189 = case shown="True" w473 {
                  tunnel: w475 -> [w476 w483]
                  tunnel: [w476 w481] -> w474
                  tunnel: [_ w478] -> w472
                  frame False {
                    n190 = One Button Dialog(message="Camera is not open") -> ()  [unwired: 1 in, 1 out]
                  }
                  frame True {
                    w488 = 0 items=["Idle", "Capturing"] ("Status")
                    n191 = property class="Camera"(reference=w483) -> (reference out=w482:refnum<k24>, error out=w479:errorcluster, "IsOpen"=w487:bool, "Status"=w489:i32)  [unwired: 1 in]
                    n192 = Equal?(x=w487, y=TRUE) -> (x = y?=w485:bool)
                    n193 = Equal?(x=w489, y=w488) -> (x = y?=w484:bool)
                    n194 = Equal?(x=w485, y=w484) -> (x = y?=w480:bool)
                    n195 = case shown="True" w480 {
                      tunnel: w482 -> [w492 w497]
                      tunnel: [w492 w498] -> w481
                      tunnel: w479 -> [w490 w495]
                      tunnel: [w490 w493] -> w478
                      frame False {
                        n196 = local write "Live"(FALSE ("Live 2")) -> ()
                      }
                      frame True {
                        n197 = flat-sequence {
                          tunnel: w497 -> [w506]
                          tunnel: [w503] -> w496
                          tunnel: w495 -> [w502]
                          tunnel: [w500] -> w494
                          frame #0 {
                            n198 = property class="Camera"(reference=w506, error in=w502) -> (reference out=w503:refnum<k24>, error out=w501:errorcluster, "AcquisitionBuffer"=w505:refnum<k24>)
                            n199 = property class="AcqBuffer"(reference=w505, error in=w501, "BufferSize"=100) -> (error out=w500:errorcluster)  [unwired: 1 out]
                          }
                        }
                        n200 = local write "Live"(TRUE ("Live")) -> ()
                        n201 = invoke class="Camera" method="StartLive"(reference=w496, error in=w494) -> (reference out=w498:refnum<k24>, error out=w493:errorcluster)  [unwired: 1 in, 1 out]
                      }
                    }
                  }
                }
              }
            }
            n202 = case shown="True" "Live start" {
              tunnel: w430 -> [w437 w441]
              tunnel: [w437 w440] -> w431
              tunnel: w426 -> [_ w439]
              tunnel: w425 -> [_ w438]
              frame False {
              }
              frame True {
                n203 = case shown="True" w439 {
                  tunnel: w441 -> [w442 w449]
                  tunnel: [w442 w447] -> w440
                  tunnel: w438 -> [_ w445]
                  frame False {
                    n204 = One Button Dialog(message="Camera is not open") -> ()  [unwired: 1 in, 1 out]
                  }
                  frame True {
                    w454 = 0 items=["Idle", "Capturing"] ("Status")
                    n205 = property class="Camera"(reference=w449, error in=w445) -> (reference out=w448:refnum<k24>, error out=w444:errorcluster, "IsOpen"=w453:bool, "Status"=w455:i32)
                    n206 = Equal?(x=w453, y=TRUE) -> (x = y?=w451:bool)
                    n207 = Equal?(x=w455, y=w454) -> (x = y?=w450:bool)
                    n208 = Equal?(x=w451, y=w450) -> (x = y?=w446:bool)
                    n209 = case shown="True" w446 {
                      tunnel: w448 -> [w457 w461]
                      tunnel: [w457 w462] -> w447
                      tunnel: w444 -> [_ w459]
                      frame False {
                        n210 = local write "Live 3"(FALSE ("Live 2")) -> ()
                      }
                      frame True {
                        n211 = flat-sequence {
                          tunnel: w461 -> [w470]
                          tunnel: [w467] -> w460
                          tunnel: w459 -> [w466]
                          tunnel: [w464] -> w458
                          frame #0 {
                            n212 = property class="Camera"(reference=w470, error in=w466) -> (reference out=w467:refnum<k24>, error out=w465:errorcluster, "AcquisitionBuffer"=w469:refnum<k24>)
                            n213 = property class="AcqBuffer"(reference=w469, error in=w465, "BufferSize"=100) -> (error out=w464:errorcluster)  [unwired: 1 out]
                          }
                        }
                        n214 = local write "Live 2"(TRUE ("Live")) -> ()
                        n215 = invoke class="Camera" method="StartLive"(reference=w460, error in=w458) -> (reference out=w462:refnum<k24>)  [unwired: 1 in, 2 out]
                      }
                    }
                  }
                }
              }
            }
          }
          event "Stream Saving On/Off", "Format", "Big TIFF On/Off", "Multi Page TIFF Size [B]": Value Change {
            n216 = event-data() -> ()  [unwired: 1 in, 6 out]
            n217 = local read "Stream Saving On/Off"() -> (w520:bool)
            n218 = Bundle("get_Item"=w517, "Event Callback"=w516, "Event Callback"=w515) -> (w514:T1)  [unwired: 1 in]
            n219 = local read "Camera Status"() -> (w527:bool)
            n220 = local read "StreamSavingPath"() -> (w522:string)
            n221 = local read "Format"() -> (w521:u8)
            n222 = local read "Multi Page TIFF Size [B]"() -> (w510:u64)
            n223 = local read "Big TIFF On/Off"() -> (w509:bool)
            n224 = case shown="True" w527 {
              tunnel: w526 -> [w532 w545]
              tunnel: [w532 w542] -> w525
              tunnel: w522 -> [w531 w541]
              tunnel: w521 -> [w530 w540]
              tunnel: w520 -> [_ w539]
              tunnel: [w531 w538] -> w519
              tunnel: [w530 w537] -> w518
              tunnel: w510 -> [w528 w536]
              tunnel: w509 -> [w529 w535]
              tunnel: [w529 w534] -> w508
              tunnel: [w528 w533] -> w507
              frame False {
              }
              frame True {
                w550 = 0 items=["Idle", "Capturing"] ("Status")
                n225 = property class="Camera"(reference=w545) -> (reference out=w543:refnum<k24>, "IsOpen"=w549:bool, "Status"=w551:i32)  [unwired: 1 in, 1 out]
                n226 = Equal?(x=w549, y=TRUE) -> (x = y?=w547:bool)
                n227 = Equal?(x=w551, y=w550) -> (x = y?=w546:bool)
                n228 = Equal?(x=w547, y=w546) -> (x = y?=w544:bool)
                n229 = case shown="True" w544 {
                  tunnel: w543 -> [w557 w572]
                  tunnel: [w557 w571] -> w542
                  tunnel: w541 -> [w555 w569]
                  tunnel: w540 -> [w554 w568]
                  tunnel: w539 -> [_ w567]
                  tunnel: [w555 w566] -> w538
                  tunnel: [w554 w565] -> w537
                  tunnel: w536 -> [w552 w564]
                  tunnel: w535 -> [w553 w563]
                  tunnel: [w553 w559] -> w534
                  tunnel: [w552 w558] -> w533
                  frame False {
                    n230 = One Button Dialog(message="Camera is not idle") -> ()  [unwired: 1 in, 1 out]
                  }
                  frame True {
                    n231 = local write "Stream Saving"(w567) -> ()
                    n232 = property class="Camera"(reference=w572) -> (reference out=w571:refnum<k24>, "AcquisitionBuffer"=w570:refnum<k24>)  [unwired: 1 in, 1 out]
                    n233 = property class="AcqBuffer"(reference=w570, "DiskStreamingRequired"=w567, "DiskStreamingSavingPath"=w569, "DiskStreamingFormat"=w568) -> (reference out=w562:refnum<k24>)  [unwired: 1 in, 1 out]
                    n234 = property class="AcqBuffer"(reference=w562, "BigTiffRequired"=w563, "MultiPageFrameSize"=w564) -> (reference out=w561:refnum<k24>)  [unwired: 1 in, 1 out]
                    n235 = property class="AcqBuffer"(reference=w561) -> (reference out=w560:refnum<k24>, "DiskStreamingSavingPath"=w566:string, "DiskStreamingFormat"=w565:u32)  [unwired: 1 in, 1 out]
                    n236 = property class="AcqBuffer"(reference=w560) -> ("BigTiffRequired"=w559:bool, "MultiPageFrameSize"=w558:u64)  [unwired: 1 in, 2 out]
                  }
                }
              }
            }
            n237 = local write "StreamSavingPath"(w519) -> ()
            n238 = local write "Big TIFF"(w508) -> ()
            n239 = local write "Multi Page TIFF Size Read"(w507) -> ()
            n240 = local write "Format"(w518) -> ()
            n241 = Unbundle(w514) -> ("get_Item"=w513:refnum<k24>, "Event Callback"=w512:refnum<k27>, "Event Callback"=w511:refnum<k27>)
          }
          event "Stream Saving On/Off 2", "Format 2", "Big TIFF On/Off 2", "Multi Page TIFF Size 2 [B]": Value Change {
            n242 = event-data() -> ()  [unwired: 1 in, 6 out]
            n243 = Bundle("get_Item"=w583, "Event Callback"=w582, "Event Callback"=w581) -> (w580:T1)  [unwired: 1 in]
            n244 = local read "Stream Saving On/Off 2"() -> (w589:bool)
            n245 = local read "StreamSavingPath 2"() -> (w588:string)
            n246 = local read "Format 2"() -> (w587:u8)
            n247 = local read "Multi Page TIFF Size 2 [B]"() -> (w576:u64)
            n248 = local read "Big TIFF On/Off 2"() -> (w575:bool)
            n249 = local read "Camera Status"() -> (w590:bool)
            n250 = case shown="True" w590 {
              tunnel: w593 -> [w598 w611]
              tunnel: [w598 w608] -> w584
              tunnel: w588 -> [w597 w607]
              tunnel: w587 -> [w596 w606]
              tunnel: w589 -> [_ w605]
              tunnel: [w597 w604] -> w586
              tunnel: [w596 w603] -> w585
              tunnel: w576 -> [w594 w602]
              tunnel: w575 -> [w595 w601]
              tunnel: [w594 w600] -> w574
              tunnel: [w595 w599] -> w573
              frame False {
              }
              frame True {
                w616 = 0 items=["Idle", "Capturing"] ("Status")
                n251 = property class="Camera"(reference=w611) -> (reference out=w609:refnum<k24>, "IsOpen"=w615:bool, "Status"=w617:i32)  [unwired: 1 in, 1 out]
                n252 = Equal?(x=w615, y=TRUE) -> (x = y?=w613:bool)
                n253 = Equal?(x=w617, y=w616) -> (x = y?=w612:bool)
                n254 = Equal?(x=w613, y=w612) -> (x = y?=w610:bool)
                n255 = case shown="True" w610 {
                  tunnel: w609 -> [w623 w638]
                  tunnel: [w623 w637] -> w608
                  tunnel: w607 -> [w621 w635]
                  tunnel: w606 -> [w620 w634]
                  tunnel: w605 -> [_ w633]
                  tunnel: [w621 w632] -> w604
                  tunnel: [w620 w631] -> w603
                  tunnel: w602 -> [w618 w627]
                  tunnel: w601 -> [w619 w626]
                  tunnel: [w618 w625] -> w600
                  tunnel: [w619 w624] -> w599
                  frame False {
                    n256 = One Button Dialog(message="Camera is not idle") -> ()  [unwired: 1 in, 1 out]
                  }
                  frame True {
                    n257 = local write "Stream Saving 2"(w633) -> ()
                    n258 = property class="Camera"(reference=w638) -> (reference out=w637:refnum<k24>, "AcquisitionBuffer"=w636:refnum<k24>)  [unwired: 1 in, 1 out]
                    n259 = property class="AcqBuffer"(reference=w636, "DiskStreamingRequired"=w633, "DiskStreamingSavingPath"=w635, "DiskStreamingFormat"=w634) -> (reference out=w630:refnum<k24>)  [unwired: 1 in, 1 out]
                    n260 = property class="AcqBuffer"(reference=w630, "BigTiffRequired"=w626, "MultiPageFrameSize"=w627) -> (reference out=w629:refnum<k24>)  [unwired: 1 in, 1 out]
                    n261 = property class="AcqBuffer"(reference=w629) -> (reference out=w628:refnum<k24>, "DiskStreamingSavingPath"=w632:string, "DiskStreamingFormat"=w631:u32)  [unwired: 1 in, 1 out]
                    n262 = property class="AcqBuffer"(reference=w628) -> ("BigTiffRequired"=w624:bool, "MultiPageFrameSize"=w625:u64)  [unwired: 1 in, 2 out]
                  }
                }
              }
            }
            n263 = local write "StreamSavingPath 2"(w586) -> ()
            n264 = local write "Format 2"(w585) -> ()
            n265 = local write "Multi Page TIFF Size Read 2"(w574) -> ()
            n266 = local write "Big TIFF 2"(w573) -> ()
            n267 = Unbundle(w580) -> ("get_Item"=w579:refnum<k24>, "Event Callback"=w578:refnum<k27>, "Event Callback"=w577:refnum<k27>)
          }
          event "Path": Value Change {
            n268 = event-data() -> ()  [unwired: 1 in, 6 out]
            n269 = local read "Camera Status"() -> (w651:bool)
            n270 = Bundle("get_Item"=w645, "Event Callback"=w644, "Event Callback"=w643) -> (w642:T1)  [unwired: 1 in]
            n271 = local read "Path"() -> (w646:path)
            n272 = case shown="True" w651 {
              tunnel: w650 -> [w652 w658]
              tunnel: [w652 w655] -> w649
              tunnel: w646 -> [_ w654]
              tunnel: w646 -> [_ w653]
              frame False {
              }
              frame True {
                w663 = 0 items=["Idle", "Capturing"] ("Status")
                n273 = property class="Camera"(reference=w658) -> (reference out=w656:refnum<k24>, "IsOpen"=w662:bool, "Status"=w664:i32)  [unwired: 1 in, 1 out]
                n274 = Equal?(x=w662, y=TRUE) -> (x = y?=w660:bool)
                n275 = Equal?(x=w664, y=w663) -> (x = y?=w659:bool)
                n276 = Equal?(x=w660, y=w659) -> (x = y?=w657:bool)
                n277 = case shown="True" w657 {
                  tunnel: w656 -> [w666 w673]
                  tunnel: [w666 w672] -> w655
                  tunnel: w654 -> [_ w669]
                  tunnel: w653 -> [_ w668]
                  frame False {
                    n278 = One Button Dialog(message="Camera is not idle") -> ()  [unwired: 1 in, 1 out]
                  }
                  frame True {
                    n279 = call <vilib>:"Check if File or Folder Exists.vi"("path"=w668) -> ("file or folder exists?"=w670:bool)  [unwired: 8 in, 2 out]
                    n280 = case shown="True" w670 {
                      tunnel: w669 -> [_ w679]
                      tunnel: ["" w676] -> w667
                      frame False {
                        n281 = One Button Dialog(message="The specified folder doesn't exist") -> ()  [unwired: 1 in, 1 out]
                      }
                      frame True {
                        # "Here we need to append \"\\\" to the path"
                        n282 = Path To String(path=w679) -> (string=w678:string)
                        n283 = Concatenate Strings(w678, "\\" ("string")) -> (w676:string)
                      }
                    }
                    n284 = property class="Camera"(reference=w673) -> (reference out=w672:refnum<k24>, "AcquisitionBuffer"=w671:refnum<k24>)  [unwired: 1 in, 1 out]
                    n285 = property class="AcqBuffer"(reference=w671, "DiskStreamingSavingPath"=w667) -> ()  [unwired: 1 in, 2 out]
                    n286 = local write "StreamSavingPath"(w667) -> ()
                  }
                }
              }
            }
            n287 = Unbundle(w642) -> ("get_Item"=w641:refnum<k24>, "Event Callback"=w640:refnum<k27>, "Event Callback"=w639:refnum<k27>)
          }
          event "Path 2": Value Change {
            n288 = event-data() -> ()  [unwired: 1 in, 6 out]
            n289 = Bundle("get_Item"=w683, "Event Callback"=w682, "Event Callback"=w681) -> (w686:T1)  [unwired: 1 in]
            n290 = local read "Path 2"() -> (w692:path)
            n291 = local read "Camera Status"() -> (w691:bool)
            n292 = case shown="True" w691 {
              tunnel: w690 -> [w693 w699]
              tunnel: [w693 w696] -> w689
              tunnel: w692 -> [_ w695]
              tunnel: w692 -> [_ w694]
              frame False {
              }
              frame True {
                w704 = 0 items=["Idle", "Capturing"] ("Status")
                n293 = property class="Camera"(reference=w699) -> (reference out=w697:refnum<k24>, "IsOpen"=w703:bool, "Status"=w705:i32)  [unwired: 1 in, 1 out]
                n294 = Equal?(x=w703, y=TRUE) -> (x = y?=w701:bool)
                n295 = Equal?(x=w705, y=w704) -> (x = y?=w700:bool)
                n296 = Equal?(x=w701, y=w700) -> (x = y?=w698:bool)
                n297 = case shown="True" w698 {
                  tunnel: w697 -> [w707 w714]
                  tunnel: [w707 w713] -> w696
                  tunnel: w695 -> [_ w710]
                  tunnel: w694 -> [_ w709]
                  frame False {
                    n298 = One Button Dialog(message="Camera is not idle") -> ()  [unwired: 1 in, 1 out]
                  }
                  frame True {
                    n299 = call <vilib>:"Check if File or Folder Exists.vi"("path"=w709) -> ("file or folder exists?"=w711:bool)  [unwired: 8 in, 2 out]
                    n300 = case shown="True" w711 {
                      tunnel: w710 -> [_ w720]
                      tunnel: ["" w717] -> w708
                      frame False {
                        n301 = One Button Dialog(message="The specified folder doesn't exist") -> ()  [unwired: 1 in, 1 out]
                      }
                      frame True {
                        # "Here we need to append \"\\\" to the path"
                        n302 = Path To String(path=w720) -> (string=w719:string)
                        n303 = Concatenate Strings(w719, "\\" ("string")) -> (w717:string)
                      }
                    }
                    n304 = property class="Camera"(reference=w714) -> (reference out=w713:refnum<k24>, "AcquisitionBuffer"=w712:refnum<k24>)  [unwired: 1 in, 1 out]
                    n305 = property class="AcqBuffer"(reference=w712, "DiskStreamingSavingPath"=w708) -> ()  [unwired: 1 in, 2 out]
                    n306 = local write "StreamSavingPath 2"(w708) -> ()
                  }
                }
              }
            }
            n307 = Unbundle(w686) -> ("get_Item"=w685:refnum<k24>, "Event Callback"=w684:refnum<k27>, "Event Callback"=w680:refnum<k27>)
          }
          event "Live stop": Value Change {
            n308 = event-data() -> ()  [unwired: 1 in, 6 out]
            n309 = local read "Camera Status"() -> (w727:bool)
            n310 = case shown="True" "Live stop" {
              tunnel: w731 -> [w756 w760]
              tunnel: [w756 w759] -> w730
              tunnel: w727 -> [_ w758]
              tunnel: [_ w757] -> w721
              frame False {
              }
              frame True {
                n311 = case shown="True" w758 {
                  tunnel: w760 -> [w762 w774]
                  tunnel: [w762 w771] -> w759
                  tunnel: [_ w763] -> w757
                  frame False {
                    n312 = One Button Dialog(message="Camera is not open") -> ()  [unwired: 1 in, 1 out]
                  }
                  frame True {
                    w769 = 1 items=["Idle", "Capturing"] ("Status")
                    n313 = property class="Camera"(reference=w774) -> (reference out=w772:refnum<k24>, error out=w764:errorcluster, "IsOpen"=w768:bool, "Status"=w770:i32)  [unwired: 1 in]
                    n314 = Equal?(x=w770, y=w769) -> (x = y?=w765:bool)
                    n315 = Equal?(x=w768, y=TRUE) -> (x = y?=w766:bool)
                    n316 = Equal?(x=w766, y=w765) -> (x = y?=w773:bool)
                    n317 = case shown="True" w773 {
                      tunnel: w772 -> [w775 w780]
                      tunnel: [w775 w779] -> w771
                      tunnel: w764 -> [_ w777]
                      tunnel: [_ w776] -> w763
                      frame False {
                      }
                      frame True {
                        n318 = invoke class="Camera" method="Stop"(reference=w780, error in=w777) -> (reference out=w779:refnum<k24>, error out=w776:errorcluster)  [unwired: 1 in, 1 out]
                        n319 = local write "Live"(FALSE ("Live 2")) -> ()
                      }
                    }
                  }
                }
              }
            }
            n320 = case shown="True" "Live stop" {
              tunnel: w726 -> [w732 w736]
              tunnel: [w732 w735] -> w725
              tunnel: w727 -> [_ w734]
              tunnel: w721 -> [_ w733]
              frame False {
              }
              frame True {
                n321 = case shown="True" w734 {
                  tunnel: w736 -> [w738 w750]
                  tunnel: [w738 w747] -> w735
                  tunnel: w733 -> [_ w740]
                  frame False {
                    n322 = One Button Dialog(message="Camera is not open") -> ()  [unwired: 1 in, 1 out]
                  }
                  frame True {
                    w745 = 1 items=["Idle", "Capturing"] ("Status")
                    n323 = property class="Camera"(reference=w750, error in=w740) -> (reference out=w748:refnum<k24>, error out=w739:errorcluster, "IsOpen"=w744:bool, "Status"=w746:i32)
                    n324 = Equal?(x=w746, y=w745) -> (x = y?=w741:bool)
                    n325 = Equal?(x=w744, y=TRUE) -> (x = y?=w742:bool)
                    n326 = Equal?(x=w742, y=w741) -> (x = y?=w749:bool)
                    n327 = case shown="True" w749 {
                      tunnel: w748 -> [w751 w755]
                      tunnel: [w751 w754] -> w747
                      tunnel: w739 -> [_ w752]
                      frame False {
                      }
                      frame True {
                        n328 = invoke class="Camera" method="Stop"(reference=w755, error in=w752) -> (reference out=w754:refnum<k24>)  [unwired: 1 in, 2 out]
                        n329 = local write "Live 2"(FALSE ("Live 2")) -> ()
                      }
                    }
                  }
                }
              }
            }
          }
          event "Uninit": Value Change {
            n330 = event-data() -> ()  [unwired: 1 in, 6 out]
            n331 = case shown="True" "Uninit" {
              tunnel: w789 -> [w802 w816]
              tunnel: [w802 w815] -> w795
              tunnel: [FALSE ("Camera Status") w813] -> w793
              tunnel: w791 -> [w800 w812]
              tunnel: [w800 w811] -> w790
              tunnel: [w799 w810] -> w788
              tunnel: w787 -> [w799 w809]
              tunnel: [w797 w808] -> w786
              tunnel: [w796 w807] -> w785
              tunnel: w784 -> [w798 w806]
              tunnel: w783 -> [w797 w805]
              tunnel: w782 -> [w796 w804]
              tunnel: [w798 w803] -> w781
              frame False {
              }
              frame True {
                n332 = local read "Camera Status"() -> (w814:bool)
                n333 = case shown="True" w814 {
                  tunnel: w816 -> [w823 w841]
                  tunnel: [w823 w840] -> w815
                  tunnel: [FALSE ("Camera Status") w839] -> w813
                  tunnel: w812 -> [w821 w838]
                  tunnel: [w821 w837] -> w811
                  tunnel: [w820 w836] -> w810
                  tunnel: w809 -> [w820 w835]
                  tunnel: [w818 w834] -> w808
                  tunnel: [w817 w833] -> w807
                  tunnel: w806 -> [w819 w832]
                  tunnel: w805 -> [w818 w831]
                  tunnel: w804 -> [w817 w830]
                  tunnel: [w819 w824] -> w803
                  frame False {
                  }
                  frame True {
                    n334 = local read "Live 2"() -> (w828:bool)
                    n335 = local read "Live"() -> (w829:bool)
                    n336 = Not(x=w829) -> (.not. x?=w826:bool)
                    n337 = Not(x=w828) -> (.not. x?=w827:bool)
                    n338 = And(x=w826, y=w827) -> (x .and. y?=w825:bool)
                    n339 = case shown="True" w825 {
                      tunnel: w841 -> [w849 w863]
                      tunnel: [w849 w862] -> w840
                      tunnel: [FALSE ("Camera Status") w861] -> w839
                      tunnel: w838 -> [w847 w860]
                      tunnel: [w847 w859] -> w837
                      tunnel: [w846 w858] -> w836
                      tunnel: w835 -> [w846 w857]
                      tunnel: [w843 w856] -> w834
                      tunnel: [w842 w855] -> w833
                      tunnel: w832 -> [w844 w853]
                      tunnel: w831 -> [w843 w852]
                      tunnel: w830 -> [w842 w851]
                      tunnel: [w844 w850] -> w824
                      frame False {
                        n340 = One Button Dialog(message="Live must be stopped to uninitialize !") -> ()  [unwired: 1 in, 1 out]
                      }
                      frame True {
                        n341 = flat-sequence {
                          tunnel: w863 -> [w873]
                          tunnel: [w872] -> w864
                          tunnel: w860 -> [w871]
                          tunnel: w857 -> [w870]
                          tunnel: [w869] -> w854
                          tunnel: w853 -> [w868]
                          tunnel: w852 -> [w867]
                          tunnel: w851 -> [w866]
                          tunnel: [w896] -> w862
                          tunnel: w864 -> [w896]
                          tunnel: [TRUE ("Camera Status")] -> w861
                          tunnel: [refnum<k27> refnum ("Event Callback")] -> w859
                          tunnel: [refnum<k27> refnum ("Event Callback")] -> w858
                          tunnel: [refnum<k27> refnum ("Event Callback")] -> w856
                          tunnel: [refnum<k27> refnum ("Event Callback")] -> w855
                          tunnel: [w889] -> w850
                          tunnel: w854 -> [w889]
                          frame #0 {
                            n342 = invoke class="Camera" method="Close"(reference=w873) -> (reference out=w872:refnum<k24>, error out=w865:errorcluster)  [unwired: 2 in, 1 out]
                            n343 = invoke class="Camera" method="Close"(reference=w868, error in=w865) -> (reference out=w869:refnum<k24>)  [unwired: 1 in, 2 out]
                            n344 = Unregister For Events(event registration refnum=w867) -> ()  [unwired: 1 in, 1 out]
                            n345 = Unregister For Events(event registration refnum=w871) -> ()  [unwired: 1 in, 1 out]
                            n346 = Unregister For Events(event registration refnum=w866) -> ()  [unwired: 1 in, 1 out]
                            n347 = Unregister For Events(event registration refnum=w870) -> ()  [unwired: 1 in, 1 out]
                          }
                          frame #1 {
                            w874 = FALSE ("Stream Saving On/Off 2")
                            w876 = u64 0 ("Multi Page TIFF Size Read")
                            w875 = FALSE ("Big TIFF 2")
                            n348 = local write "Camera Status"(FALSE ("Camera Status")) -> ()
                            n349 = control-ref of="Trigger Out Behaviour 2"() -> (w877:refnum<vi>)
                            n350 = control-ref of="Trigger In Behaviour 2"() -> (w880:refnum<vi>)
                            n351 = control-ref of="Trigger Out Behaviour"() -> (w887:refnum<vi>)
                            n352 = control-ref of="Trigger In Behaviour"() -> (w888:refnum<vi>)
                            n353 = property class="CmbBox"(reference=w888, "Value"="", "Strings[]"=string[] [] ("Strings []")) -> ()  [unwired: 1 in, 2 out]
                            n354 = property class="CmbBox"(reference=w887, "Value"="", "Strings[]"=string[] [] ("Strings []")) -> ()  [unwired: 1 in, 2 out]
                            n355 = property class="CmbBox"(reference=w877, "Value"="", "Strings[]"=string[] [] ("Strings []")) -> ()  [unwired: 1 in, 2 out]
                            n356 = property class="CmbBox"(reference=w880, "Value"="", "Strings[]"=string[] [] ("Strings []")) -> ()  [unwired: 1 in, 2 out]
                            n357 = local write "Stream Saving On/Off 2"(w874) -> ()
                            n358 = local write "Stream Saving On/Off"(w874) -> ()
                            n359 = local write "Multi Page TIFF Size [B]"(w876) -> ()
                            n360 = local write "Multi Page TIFF Size 2 [B]"(w876) -> ()
                            n361 = local write "Big TIFF 2"(w875) -> ()
                            n362 = local write "Big TIFF On/Off"(w875) -> ()
                            n363 = local write "Big TIFF On/Off 2"(w875) -> ()
                            n364 = local write "Big TIFF"(w875) -> ()
                            n365 = local write "Multi Page TIFF Size Read 2"(w876) -> ()
                            n366 = local write "Multi Page TIFF Size Read"(w876) -> ()
                          }
                        }
                      }
                    }
                  }
                }
              }
            }
          }
        }
      }
    }
    frame #2 {
      # "Live state SR"
      # "Callback SR"
      # "Camera SR"
      # "Live state SR"
      # "Callback SR"
      # "Camera SR"
      n367 = invoke class="Library" method="Release"(reference=w898) -> (reference out=w899:refnum<k24>)  [unwired: 2 in, 2 out]
      n368 = Wait (ms)(milliseconds to wait=u32 100) -> ()  [unwired: 1 out]
      n369 = Close Reference(reference=w899) -> ()  [unwired: 1 in, 1 out]
    }
    frame #3 {
      n370 = invoke class="GC" method="Collect"() -> ()  [unwired: 3 in, 3 out]
    }
  }
  n371 = local write "Camera Status"(FALSE ("Camera Status")) -> ()
  n372 = local write "Stream Saving On/Off 2"(FALSE ("Raw On/Off")) -> ()
  n373 = local write "Stream Saving On/Off"(FALSE ("Raw On/Off")) -> ()
  n374 = local write "Format 2"(u8 0 ("Format 2")) -> ()
  n375 = local write "Format"(u8 0 ("Tiff==0 Raw==1")) -> ()
  n376 = local write "Path"(path "" ("Path")) -> ()
  n377 = local write "Path 2"(path "" ("Path 2")) -> ()
  "Stream Saving" <- FALSE ("Display")
  "StreamSavingPath" <- "" ("StreamSavingPath")
  "Disk Streaming Queue Size" <- w7
  "Dropped Frames" <- w7
  "Buffer Index" <- w7
  "Available Ram" <- w7
  "Stream Saving 2" <- FALSE ("Display")
  "StreamSavingPath 2" <- "" ("StreamSavingPath 2")
  "Buffer Index 2" <- w2
  "Dropped Frames 2" <- w2
  "Disk Streaming Queue Size 2" <- w2
